vi "utility_panel_single_axis.vi"() -> ()   [LabVIEW 2014]
doc: "This VI is to serve as (1) an example of how one might incorporate the many features of the stepper motor control API into their own application and (2) allows the user to take control of their hardware for demonstration and or troubleshooting purposes. Tips and descriptions have been applied to each control on the interface. Click the HELP button to see more detailed descriptions of each control and their function.\n\nProduced By:\n\nChristopher Lemieux\nKod Integrations, LLC\n4835 Marianne Drive\nMount Airy, MD 21771\nhttp://www.kodintegrations.com\nemail: clemieux@kodintegrations.com\nphone: (240) 687-1288"
uses:
  common/controls/motor_status.ctl
  common/controls/utility_actions.ctl
  classes/Controller/_Controller.lvclass/_Controller.ctl
  common/controls/linear_direction.ctl
  common/controls/movement_item.ctl
  common/controls/axis.ctl
  common/controls/digital_output.ctl
  common/controls/polarity_item.ctl
  common/controls/polarity.ctl
  common/controls/move_mode.ctl
  common/controls/error_actions.ctl
  classes/Controller/_Controller.lvclass
  libraries/common.lvlib
panel:
  in  "help":bool
  out "status (disp)":T1(ring)=enum."CONST"
  out "Current Position (display)":i32=100 min=1 max=5000
  out "date":string
  out "power_led":bool
  in  "on/off":bool
  out "dig_ins":T2
  out "status":T3=enum."CONST"
  in  "jog_to_pos":i32 caption="Jog To Value"
  in  "move_to":bool caption="Jog To..."
  in  "home_neg":bool caption="Home (-)"
  in  "home_pos":bool caption="Home (+)"
  in  "clear":bool caption="Clear Error Codes"
  in  "Tab Control":T4(tab)
  in  "move_mode":enum32{"Abs:", "Inc:"}(radio)
  in  "position_val_set":bool
  out "position_val_actual":i32=100 min=1 max=5000
  in  "position_val_desired":i32
  in  "zero":bool
  in  "demo_start":bool
  in  "pos_3":i32
  in  "pos_2":i32
  in  "pos_1":i32
  in  "accel_set":bool
  out "accel_act":i32=100 min=1 max=5000
  in  "accel":i32=100 min=10 max=1000
  in  "low_speed_set":bool
  in  "high_speed_set":bool
  out "low_speed_act":i32=100 min=100 max=490550
  out "high_speed_act":i32=1 min=1 max=400000
  in  "low_speed":i32=100 min=100 max=490550
  in  "high_speed":i32=50 min=1 max=400000 step=1
  in  "dig_outs":T5
  out "actual_amp":i32
  in  "polarities":T6
  in  "cgh_id":bool
  in  "new_id":string
  in  "run_amp_set":bool
  in  "idle_amp_set":bool
  out "running_amp_act":i32
  out "idle_amp_act":i32
  in  "running_amp":i32=50 min=50 max=2500
  in  "idle_amp":i32=50 min=50 max=2500 step=1
  out "response":string
  out "firmware_ver":string
  out "dev_id":string
  out "prod_id":string
  in  "terminate":bool
  in  "jog_neg":bool caption="Jog (-)"
  in  "jog_pos":bool caption="Jog (+)"
  in  "imm_stop":bool caption="Stop Immediately"
  in  "slow_stop":bool caption="Stop Slowly"
  in  "raw_cmd":string
  in  "write_cmd":bool
  out "error out":errorcluster
  in  "error in (no error)":errorcluster
  # "Firmware:"
  # "Prod ID:"
  # "Dev ID:"
  # "Digital Inputs"
  # "Current Position"
  # "Status:"
  # "Current State"
  # "Mode"
  # "Speed Settings (pps)"
  # "set"
  # "(actual)"
  # "High"
  # "Low"
  # "Acceleration (ms)"
  # "set"
  # "(actual)"
  # "Accel"
  # "Demonstration"
  # "Zero First?"
  # "Position (1)"
  # "Position (2)"
  # "Position (3)"
  # "Position (ticks)"
  # "set"
  # "(actual)"
  # "new"
  # "Current Settings (mA)"
  # "set"
  # "(actual)"
  # "Idle"
  # "Run"
  # "[actual at runtime]"
  # "Polarity Settings:"
  # "Device ID:"
  # "Digital Outputs:"
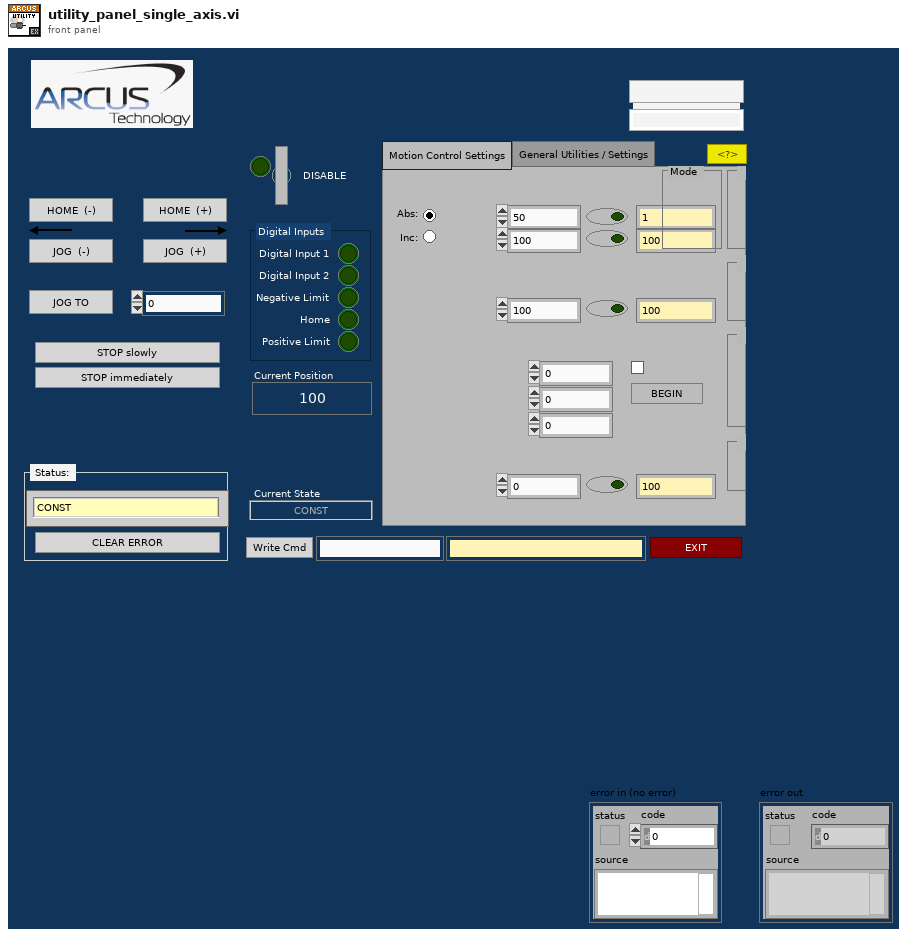
[diagram p1: front panel]
types:
  T1 = enum16{"IDLE", "CONST", "ACCEL", "DECEL", "HOME_SWITCH", "-LIMIT_SWITCH", "+LIMIT_SWITCH", "-LIMIT_ERR", "+LIMIT_ERR", "COMM_TIMEOUT", "ALARM_INPUT", "ALARM_ERROR", "TOC_TIMEOUT_STATUS", "LATCH_INPUT_STATUS", "Z_INDEX_STATUS"}
  T2 = cluster{"Digital Input 1":bool, "Digital Input 2":bool, "Negative Limit":bool, "Home":bool, "Positive Limit":bool}
  T3 = typedef "common.lvlib/motor_status.ctl" = enum16{"IDLE", "CONST", "ACCEL", "DECEL", "HOME_SWITCH", "-LIMIT_SWITCH", "+LIMIT_SWITCH", "-LIMIT_ERR", "+LIMIT_ERR", "COMM_TIMEOUT", "ALARM_INPUT", "ALARM_ERROR", "TOC_TIMEOUT_STATUS", "LATCH_INPUT_STATUS", "Z_INDEX_STATUS"}
  T4 = enum32{"Motion Control Settings", "General Utilities / Settings"}
  T5 = cluster{"Digital Output 1":bool, "Digital Output 2":bool}
  T6 = cluster{"Direction":bool, "Limit":bool, "Home":bool, "Digital Output":bool, "Digital Input":bool, "Enable Output":bool, "Jump On Error":bool}
  T7 = typedef "common.lvlib/utility_actions.ctl" = enum16{"------- unused -------", "about", "checkModel", "clearError", "closeRef", "demo", "getAcceleration", "getActualCurrentVal", "getDeviceId", "getDeviceList", "getDigInputs", "getDigOutputs", "getDriverPowerStatus", "getFirmwareVer", "getHighSpeed", "getIdleCurrent", "getLowSpeed", "getMode", "getPolarity", "getPosition", "getProductId", "getRunCurrent", "getStatus", "homeMotorNeg", "homeMotorPos", "initialize", "jogConstNeg", "jogConstPos", "moveToPos", "openRef", "pause", "powerOFF", "powerON", "processEvents", "rawCmd", "setAcceleration", "setDeviceId", "setDigOutput", "setHighSpeed", "setLowSpeed", "setPolarity", "setPosition", "setRunCurrent", "setIdleCurrent", "setMode", "setTimeOuts", "stopImmediately", "stopSlowly", "storeToFlashMem", "updatePanelItems", "validateDemoPos", "validatePos", "waitUntilDone", "zeroPosition"}
  T8 = typedef "common.lvlib/error_actions.ctl" = enum16{"clearBuff", "closeRef", "nodeErr", "noDeviceInfo", "noDevices", "openRef", "sendReceive", "setTimeouts", "unknown"}
  T9 = typedef "common.lvlib/linear_direction.ctl" = enum16{"POS (+)", "NEG (-)"}
  T10 = typedef "common.lvlib/movement_item.ctl" = cluster{"axis":T11, "target":i32}
  T11 = typedef "common.lvlib/axis.ctl" = enum16{"X", "Y", "Z", "U"}
  T12 = typedef "common.lvlib/digital_output.ctl" = enum16{"DIG_OUT_1", "DIG_OUT_2", "DIG_OUT_3", "DIG_OUT_4", "DIG_OUT_5", "DIG_OUT_6", "DIG_OUT_7", "DIG_OUT_8"}
  T13 = typedef "common.lvlib/polarity_item.ctl" = cluster{"item":T14, "status":bool}
  T14 = typedef "common.lvlib/polarity.ctl" = enum16{"DIRECTION", "LIMIT", "HOME", "DIG_OUT", "DIG_IN", "ENABLE_OUT", "JUMP_ERR", "LATCH", "Z-CHAN_INDEX", "ENCODER_DECODING:1X", "ENCODER_DECODING:2X", "ENCODER_DECODING:4X", "ALARM", "STANDALONE_ERR", "-", "<reserved/nc>"}
  T15 = typedef "common.lvlib/move_mode.ctl" = enum16{"ABSOLUTE", "INCREMENTAL"}
  T16 = typedef "common.lvlib/models.ctl" = enum16{"<unrecognized>", "ACE-SDC", "ACE-SDE", "ACE-SXC", "ACE-SXE", "DMX-CAN", "DMX-J-SA", "DMX-K-SA", "DMX-UMD", "PMX-2ED-SA", "PMX-2EX-SA", "PMX-4CX-SA", "PMX-4EX-SA"}
  T17 = typedef "common.lvlib/digital_input_item.ctl" = cluster{"item":T18, "status":bool}
  T18 = typedef "common.lvlib/digital_input.ctl" = enum16{"DIG_IN_1", "DIG_IN_2", "DIG_IN_3", "DIG_IN_4", "DIG_IN_5", "DIG_IN_6", "DIG_IN_7", "DIG_IN_8", "NEG_LIMIT", "HOME", "POS_LIMIT"}
  T19 = cluster{"[0]":bool, "[1]":bool, "[2]":bool, "[3]":bool, "[4]":bool}
  T20 = typedef "common.lvlib/digital_output_item.ctl" = cluster{"item":T12, "status":bool}
  T21 = cluster{"[0]":bool, "[1]":bool, "[2]":bool, "[3]":bool, "[4]":bool, "[5]":bool, "[6]":bool}
  T22 = typedef "common.lvlib/complete_motor_state.ctl" = cluster{"X":T23, "Y":T23, "Z":T23, "U":T23, "buffer_enabled?":bool, "buffer_start":i32, "buffer_end":i32, "avail_buffer":i32, "move_mode":T15}
  T23 = typedef "common.lvlib/single_axis_state.ctl" = cluster{"motion_state":T3, "other_states":T3[]}
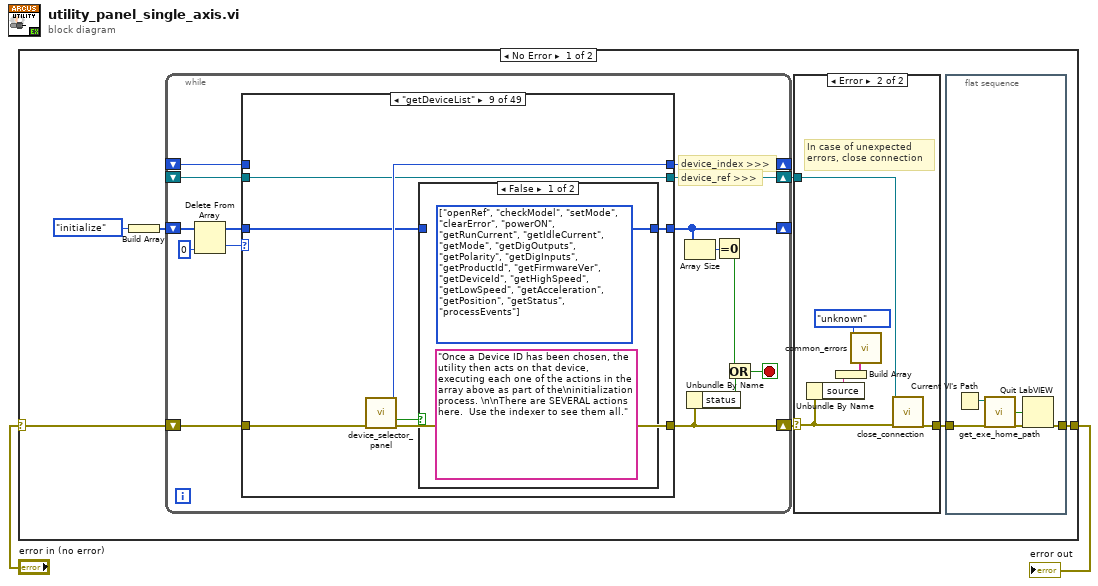
[diagram p0: block diagram]
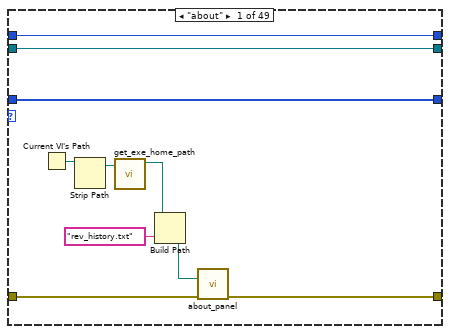
[diagram p3: hidden frame]
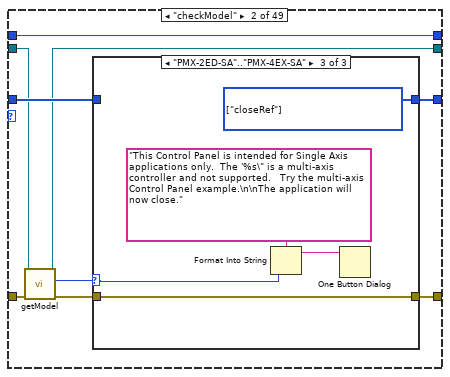
[diagram p4: hidden frame]
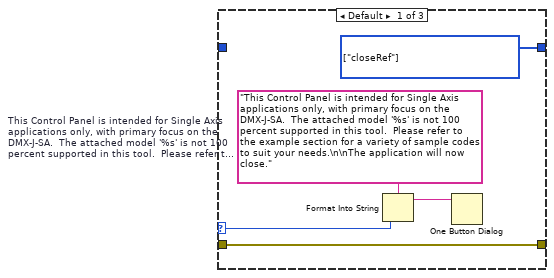
[diagram p5: hidden frame]
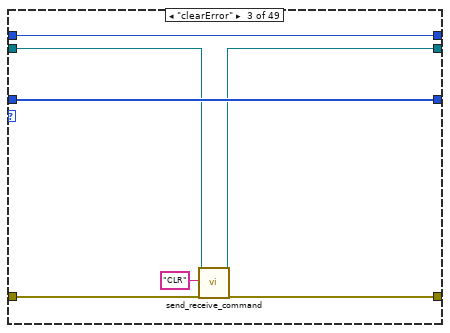
[diagram p7: hidden frame]
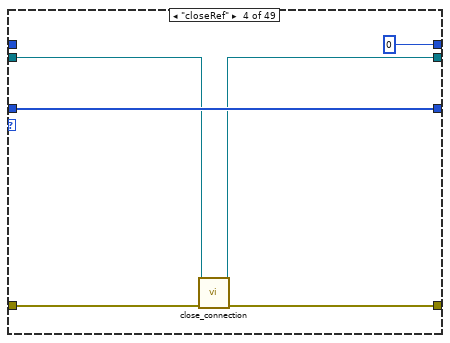
[diagram p8: hidden frame]
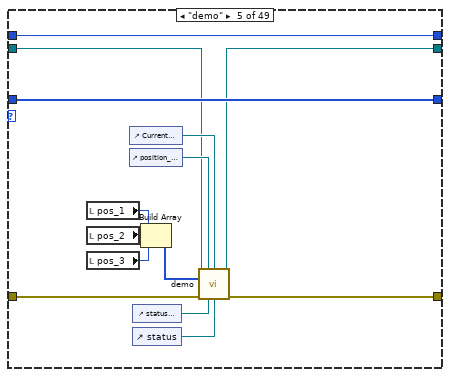
[diagram p9: hidden frame]
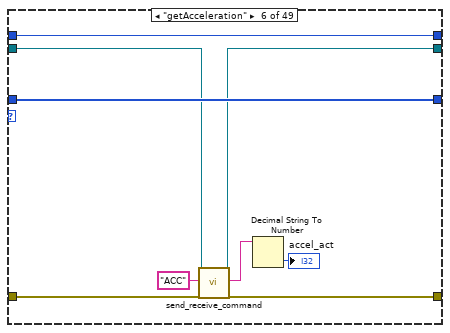
[diagram p10: hidden frame]
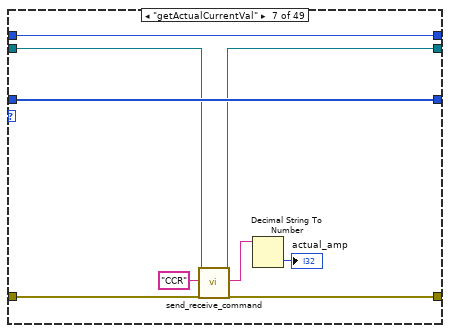
[diagram p11: hidden frame]
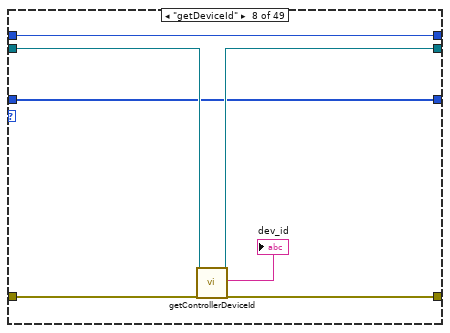
[diagram p12: hidden frame]
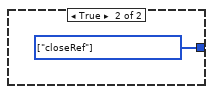
[diagram p13: hidden frame]
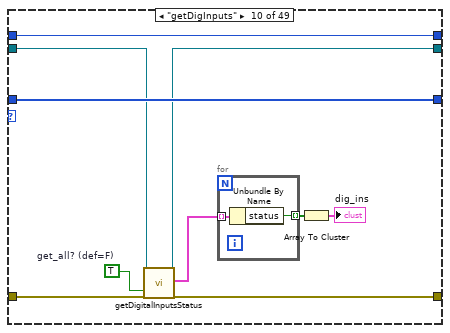
[diagram p14: hidden frame]
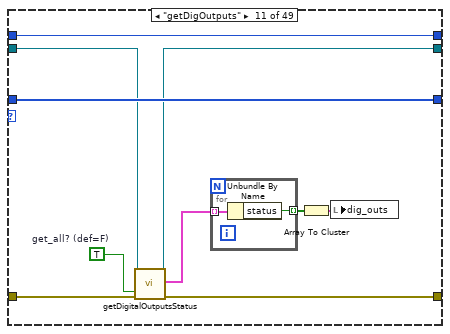
[diagram p15: hidden frame]
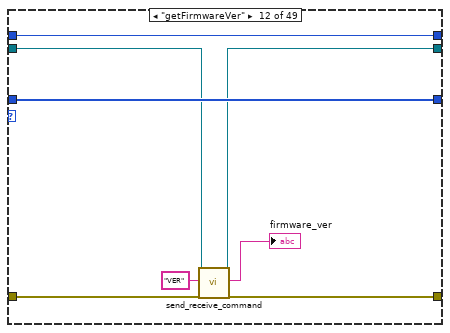
[diagram p16: hidden frame]
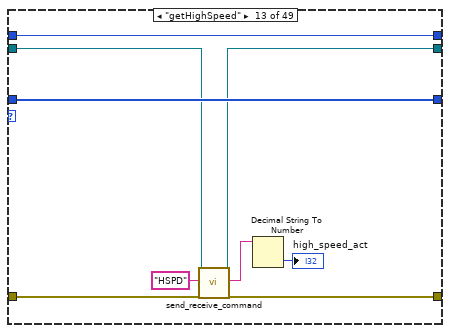
[diagram p17: hidden frame]
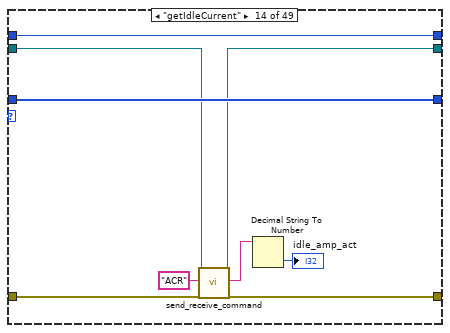
[diagram p18: hidden frame]
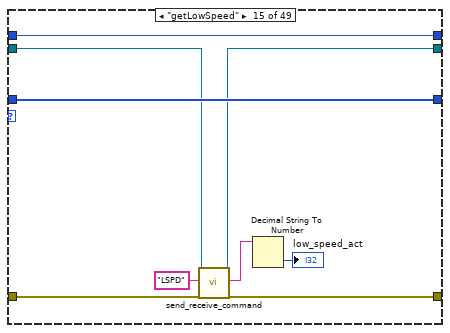
[diagram p19: hidden frame]
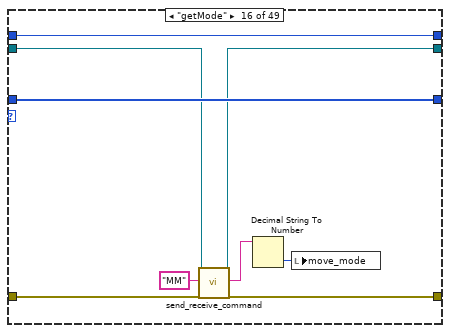
[diagram p20: hidden frame]
diagram:
  n1 = case shown="No Error" "error in (no error)" {
    selector: "error in (no error)" -> [w5 w624]
    tunnel: [w3 w624] -> w1
    frame No Error {
      n2 = Build Array(utility_actions."initialize" ("Enum")) -> (w8:T7[])
      n3 = while {
        shift-right: [w29] -> _
        shift-left: w8 -> [w34]
        shift-right: [w24] -> w7
        shift-left: w5 -> [w30]
        shift-right: [w23] -> w6
        shift-left: _ -> [w22]
        shift-right: [w21] -> _
        shift-left: _ -> [w20]
        stop <- w25 stop-if-true
        # "device_index >>>"
        # "device_ref >>>"
        n4 = Delete From Array(array=w34, index=0) -> (deleted portion=w32:T7, array with subset deleted=w31:T7[])  [unwired: 1 in]
        n5 = case shown="\"getDeviceList\"" w32 {
          tunnel: w31 -> [w44 w51 w72 w78 w88 w101 w110 w111 w119 w136 w148 w158 w167 w176 w185 w194 w203 w212 w220 w229 w237 w245 w253 _ w268 w276 w287 w295 w303 w311 w314 w416 w427 w439 w459 w470 w481 w491 w505 w516 w527 w537 w548 w556 w563 w567 w575 w601 w622]
          tunnel: [w44 w50 w72 w78 w88 w101 w110 w111 w118 w136 w148 w158 w167 w176 w185 w194 w203 w212 w220 w229 w237 w245 w253 w258 w268 w276 w286 w295 w303 w311 w315 w416 w426 w438 w458 w469 w480 w491 w504 w515 w526 w536 w548 w556 w563 w565 w571 w598 w621] -> w29
          tunnel: w30 -> [w41 w52 w70 w77 w87 w99 w108 w117 w124 w131 w146 w156 w165 w174 w183 w192 w201 w210 w218 w227 w235 w242 w250 w260 w265 w273 w284 w294 w300 w308 w318 w417 w425 w437 w455 w468 w479 w487 w503 w514 w525 w532 w546 w554 w561 w564 w572 w599 w620]
          tunnel: [w40 w45 w69 w76 w84 w98 w107 w116 w123 w130 w143 w155 w164 w173 w182 w191 w199 w209 w217 w226 w234 w241 w249 w260 w264 w272 w283 w293 w299 w307 w317 errorcluster {"status"=FALSE, "code"=0, "source"=""} w424 w433 w446 w467 w478 w486 w502 w513 w524 w533 w545 w553 w560 w564 w573 w600 w619] -> w24
          tunnel: [w42 w47 w67 w73 w79 w96 w105 w114 w121 w128 w144 w153 w162 w171 w180 w189 w200 w208 w215 w224 w233 w239 w247 w254 w262 w270 w281 w291 w298 w306 w312 w411 w422 w435 w449 w465 w476 w484 w500 w511 w522 w530 w543 w551 w558 w568 w589 w606 w617] -> w23
          tunnel: w22 -> [w42 w48 w68 w75 w80 w97 w106 w115 w121 w129 w145 w154 w163 w172 w181 w190 w196 w206 w216 w225 w232 w240 w248 w254 w263 w271 w282 _ w296 w304 w312 w412 w423 w436 w454 w466 w477 w485 w501 w512 w523 w531 w544 w552 w559 w568 w589 w606 w618]
          tunnel: [w43 w53 w71 0 ("reference (out)") w89 w100 w109 w113 w122 w135 w147 w157 w166 w175 w184 w193 w202 w211 w219 w228 w236 w244 w252 0 ("index") w267 w275 w288 w292 w302 w310 w313 w413 w428 w440 w460 w471 w482 w492 w506 w517 w528 w538 w547 w555 w562 w569 w590 w607 w623] -> w21
          tunnel: w20 -> [w43 w53 w71 _ w89 w100 w109 w113 _ w135 w147 w157 w166 w175 w184 w193 w202 w211 w219 w228 w236 w244 w252 _ w267 w275 w288 w292 w302 w310 w313 w413 w428 w440 w460 w471 w482 w492 w506 w517 w528 w538 w547 w555 w562 w569 w590 w607 w623]
          frame "about" {
            n6 = Current VI's Path() -> (path=w37:path)
            n7 = Strip Path(path=w37) -> (stripped path=w36:path)  [unwired: 1 out]
            n8 = call "get_exe_home_path.vi"("home_path"=w36) -> ("actual_home_path"=w35:path)  [unwired: 6 in, 1 out]
            n9 = Build Path(base path=w35, name or relative path="rev_history.txt") -> (appended path=w38:path)
            n10 = call "about_panel.vi"("rev_history_filepath"=w38, "error in (no error)"=w41) -> ("error out"=w40:errorcluster)  [unwired: 13 in]
          }
          frame "checkModel" {
            n11 = call "getModel.vi"("error in (no error)"=w52, "reference (in)"=w48) -> ("error out"=w46:errorcluster, "model"=w49:T16, "reference (out)"=w47:refnum<class "_Controller.lvclass">)  [unwired: 7 in]
            n12 = case shown="\"PMX-2ED-SA\"..\"PMX-4EX-SA\"" w49 {
              selector: w49 -> [w55 _ w62]
              tunnel: w51 -> [_ w60 _]
              tunnel: [w54 w60 w64] -> w50
              tunnel: [w58 w59 w65] -> w45
              tunnel: w46 -> [w58 w59 w65]
              frame Default {
                w57 = "This Control Panel is intended for Single Axis applications only, with primary focus on the DMX-J-SA.  The attached model '%s' is not 100 percent supported in this tool.  Please refer to the example section for a variety of sample codes to suit your needs.\n\nThe application will now close."  # This Control Panel is intended for Single Axis applications only, with primary focus on the DMX-J-SA.  The attached model '%s' is not 100 percent supported in this tool.  Please refer to the example section for a variety of sample codes to suit your needs.  The application will now close.
                w54 = T7[] [enum."closeRef"] items=["------- unused -------", "about", "checkModel", "clearError", "closeRef", "demo", "getAcceleration", "getActualCurrentVal", "getDeviceId", "getDeviceList", "getDigInputs", "getDigOutputs", "getDriverPowerStatus", "getFirmwareVer", "getHighSpeed", "getIdleCurrent", "getLowSpeed", "getMode", "getPolarity", "getPosition", "getProductId", "getRunCurrent", "getStatus", "homeMotorNeg", "homeMotorPos", "initialize", "jogConstNeg", "jogConstPos", "moveToPos", "openRef", "pause", "powerOFF", "powerON", "processEvents", "rawCmd", "setAcceleration", "setDeviceId", "setDigOutput", "setHighSpeed", "setLowSpeed", "setPolarity", "setPosition", "setRunCurrent", "setIdleCurrent", "setMode", "setTimeOuts", "stopImmediately", "stopSlowly", "storeToFlashMem", "updatePanelItems", "validateDemoPos", "validatePos", "waitUntilDone", "zeroPosition"] ("actions")
                n13 = Format Into String(format string=w57, w55) -> (resulting string=w56:string)  [unwired: 2 in, 1 out]
                n14 = One Button Dialog(message=w56) -> ()  [unwired: 1 in, 1 out]
              }
              frame "DMX-J-SA" {
                # "fully supported"
              }
              frame "PMX-2ED-SA".."PMX-4EX-SA" {
                w64 = T7[] [enum."closeRef"] items=["------- unused -------", "about", "checkModel", "clearError", "closeRef", "demo", "getAcceleration", "getActualCurrentVal", "getDeviceId", "getDeviceList", "getDigInputs", "getDigOutputs", "getDriverPowerStatus", "getFirmwareVer", "getHighSpeed", "getIdleCurrent", "getLowSpeed", "getMode", "getPolarity", "getPosition", "getProductId", "getRunCurrent", "getStatus", "homeMotorNeg", "homeMotorPos", "initialize", "jogConstNeg", "jogConstPos", "moveToPos", "openRef", "pause", "powerOFF", "powerON", "processEvents", "rawCmd", "setAcceleration", "setDeviceId", "setDigOutput", "setHighSpeed", "setLowSpeed", "setPolarity", "setPosition", "setRunCurrent", "setIdleCurrent", "setMode", "setTimeOuts", "stopImmediately", "stopSlowly", "storeToFlashMem", "updatePanelItems", "validateDemoPos", "validatePos", "waitUntilDone", "zeroPosition"] ("actions")
                n15 = Format Into String(format string="This Control Panel is intended for Single Axis applications only.  The '%s\" is a multi-axis controller and not supported.   Try the multi-axis Control Panel example.\n\nThe application will now close.", w62) -> (resulting string=w61:string)  [unwired: 2 in, 1 out]
                n16 = One Button Dialog(message=w61) -> ()  [unwired: 1 in, 1 out]
              }
            }
          }
          frame "clearError" {
            n17 = call "send_receive_command.vi"("reference (in)"=w68, "ASCII Command (in)"="CLR", "error in (no error)"=w70) -> ("reference (out)"=w67:refnum<class "_Controller.lvclass">, "error out"=w69:errorcluster)  [unwired: 12 in, 3 out]
          }
          frame "closeRef" {
            n18 = call "close_connection.vi"("reference (in)"=w75, "error in (no error)"=w77) -> ("reference (out)"=w73:refnum<class "_Controller.lvclass">, "error out"=w76:errorcluster)  [unwired: 16 in]
          }
          frame "demo" {
            n19 = local read "pos_1"() -> (w91:i32)
            n20 = local read "pos_2"() -> (w90:i32)
            n21 = local read "pos_3"() -> (w92:i32)
            n22 = control-ref of="Current Position (display)"() -> (w83:refnum<vi>)
            n23 = control-ref of="position_val_actual"() -> (w86:refnum<vi>)
            n24 = control-ref of="status (disp)"() -> (w82:refnum<vi>)
            n25 = control-ref of="status"() -> (w81:refnum<vi>)
            n26 = Build Array(w91, w90, w92) -> (w85:i32[])
            n27 = call "demo.vi"("reference (in)"=w80, "position ref"=w86, "position (large) ref"=w83, "positions"=w85, "error in (no error)"=w87, "status (display) ref"=w82, "status ref"=w81) -> ("reference (out)"=w79:refnum<class "_Controller.lvclass">, "error out"=w84:errorcluster)  [unwired: 7 in]
          }
          frame "getAcceleration" {
            n28 = call "send_receive_command.vi"("reference (in)"=w97, "ASCII Command (in)"="ACC", "error in (no error)"=w99) -> ("reference (out)"=w96:refnum<class "_Controller.lvclass">, "response (out)"=w94:string, "error out"=w98:errorcluster)  [unwired: 12 in, 2 out]
            n29 = Decimal String To Number(string=w94) -> (number=→"accel_act":i32)  [unwired: 2 in, 1 out]
          }
          frame "getActualCurrentVal" {
            n30 = call "send_receive_command.vi"("reference (in)"=w106, "ASCII Command (in)"="CCR", "error in (no error)"=w108) -> ("reference (out)"=w105:refnum<class "_Controller.lvclass">, "response (out)"=w104:string, "error out"=w107:errorcluster)  [unwired: 12 in, 2 out]
            n31 = Decimal String To Number(string=w104) -> (number=→"actual_amp":i32)  [unwired: 2 in, 1 out]
          }
          frame "getDeviceId" {
            n32 = call "getControllerDeviceId.vi"("reference (in)"=w115, "error in (no error)"=w117) -> ("reference (out)"=w114:refnum<class "_Controller.lvclass">, "device_id (out)"=→"dev_id":string, "error out"=w116:errorcluster)  [unwired: 15 in]
          }
          frame "getDeviceList" {
            n33 = call "device_selector_panel.vi"("error in (no error)"=w124) -> ("index"=w122:i32, "cancel?"=w120:bool, "error out"=w123:errorcluster)  [unwired: 10 in, 2 out]
            n34 = case shown="False" w120 {
              tunnel: w119 -> [_ _]
              tunnel: [w125 w126] -> w118
              frame False {
                (unwired) "Once a Device ID has been chosen, the utility then acts on that device, executing each one of the actions in the array above as part of the\ninitialization process. \n\nThere are SEVERAL actions here.  Use the indexer to see them all."
                w125 = T7[] [enum."openRef", enum."checkModel", enum."setMode", enum."clearError", enum."powerON", enum."getRunCurrent", enum."getIdleCurrent", enum."getMode", enum."getDigOutputs", enum."getPolarity", enum."getDigInputs", enum."getProductId", enum."getFirmwareVer", enum."getDeviceId", enum."getHighSpeed", enum."getLowSpeed", enum."getAcceleration", enum."getPosition", enum."getStatus", enum."processEvents"] items=["------- unused -------", "about", "checkModel", "clearError", "closeRef", "demo", "getAcceleration", "getActualCurrentVal", "getDeviceId", "getDeviceList", "getDigInputs", "getDigOutputs", "getDriverPowerStatus", "getFirmwareVer", "getHighSpeed", "getIdleCurrent", "getLowSpeed", "getMode", "getPolarity", "getPosition", "getProductId", "getRunCurrent", "getStatus", "homeMotorNeg", "homeMotorPos", "initialize", "jogConstNeg", "jogConstPos", "moveToPos", "openRef", "pause", "powerOFF", "powerON", "processEvents", "rawCmd", "setAcceleration", "setDeviceId", "setDigOutput", "setHighSpeed", "setLowSpeed", "setPolarity", "setPosition", "setRunCurrent", "setIdleCurrent", "setMode", "setTimeOuts", "stopImmediately", "stopSlowly", "storeToFlashMem", "updatePanelItems", "validateDemoPos", "validatePos", "waitUntilDone", "zeroPosition"] ("actions")
              }
              frame True {
                w126 = T7[] [enum."closeRef"] items=["------- unused -------", "about", "checkModel", "clearError", "closeRef", "demo", "getAcceleration", "getActualCurrentVal", "getDeviceId", "getDeviceList", "getDigInputs", "getDigOutputs", "getDriverPowerStatus", "getFirmwareVer", "getHighSpeed", "getIdleCurrent", "getLowSpeed", "getMode", "getPolarity", "getPosition", "getProductId", "getRunCurrent", "getStatus", "homeMotorNeg", "homeMotorPos", "initialize", "jogConstNeg", "jogConstPos", "moveToPos", "openRef", "pause", "powerOFF", "powerON", "processEvents", "rawCmd", "setAcceleration", "setDeviceId", "setDigOutput", "setHighSpeed", "setLowSpeed", "setPolarity", "setPosition", "setRunCurrent", "setIdleCurrent", "setMode", "setTimeOuts", "stopImmediately", "stopSlowly", "storeToFlashMem", "updatePanelItems", "validateDemoPos", "validatePos", "waitUntilDone", "zeroPosition"] ("actions")
              }
            }
          }
          frame "getDigInputs" {
            w132 = TRUE  # get_all? (def=F)
            n35 = call "getDigitalInputsStatus.vi"("Controller in"=w129, "get_all? (def=F)"=w132, "error in (no error)"=w131) -> ("Controller out"=w128:refnum<class "_Controller.lvclass">, "di_items"=w127:T17[], "error out"=w130:errorcluster)  [unwired: 12 in, 2 out]
            n36 = for {
              tunnel: w127 -> [w138] mode=indexing
              tunnel: [w137] -> w134 mode=indexing
              n37 = Unbundle By Name(w138) -> ("status"=w137:bool)
            }
            n38 = Array To Cluster(array=w134) -> (cluster=→"dig_ins":T19)
          }
          frame "getDigOutputs" {
            w139 = TRUE  # get_all? (def=F)
            n39 = call "getDigitalOutputsStatus.vi"("Controller in"=w145, "get_all? (def=F)"=w139, "error in (no error)"=w146) -> ("Controller out"=w144:refnum<class "_Controller.lvclass">, "do_items"=w142:T20[], "error out"=w143:errorcluster)  [unwired: 12 in, 2 out]
            n40 = for {
              tunnel: w142 -> [w150] mode=indexing
              tunnel: [w149] -> w141 mode=indexing
              n41 = Unbundle By Name(w150) -> ("status"=w149:bool)
            }
            n42 = Array To Cluster(array=w141) -> (cluster=w140:cluster{"[0]":bool, "[1]":bool})
            n43 = local write "dig_outs"(w140) -> ()
          }
          frame "getFirmwareVer" {
            n44 = call "send_receive_command.vi"("reference (in)"=w154, "ASCII Command (in)"="VER", "error in (no error)"=w156) -> ("reference (out)"=w153:refnum<class "_Controller.lvclass">, "response (out)"=→"firmware_ver":string, "error out"=w155:errorcluster)  [unwired: 12 in, 2 out]
          }
          frame "getHighSpeed" {
            n45 = call "send_receive_command.vi"("reference (in)"=w163, "ASCII Command (in)"="HSPD", "error in (no error)"=w165) -> ("reference (out)"=w162:refnum<class "_Controller.lvclass">, "response (out)"=w161:string, "error out"=w164:errorcluster)  [unwired: 12 in, 2 out]
            n46 = Decimal String To Number(string=w161) -> (number=→"high_speed_act":i32)  [unwired: 2 in, 1 out]
          }
          frame "getIdleCurrent" {
            n47 = call "send_receive_command.vi"("reference (in)"=w172, "ASCII Command (in)"="ACR", "error in (no error)"=w174) -> ("reference (out)"=w171:refnum<class "_Controller.lvclass">, "response (out)"=w170:string, "error out"=w173:errorcluster)  [unwired: 12 in, 2 out]
            n48 = Decimal String To Number(string=w170) -> (number=→"idle_amp_act":i32)  [unwired: 2 in, 1 out]
          }
          frame "getLowSpeed" {
            n49 = call "send_receive_command.vi"("reference (in)"=w181, "ASCII Command (in)"="LSPD", "error in (no error)"=w183) -> ("reference (out)"=w180:refnum<class "_Controller.lvclass">, "response (out)"=w179:string, "error out"=w182:errorcluster)  [unwired: 12 in, 2 out]
            n50 = Decimal String To Number(string=w179) -> (number=→"low_speed_act":i32)  [unwired: 2 in, 1 out]
          }
          frame "getMode" {
            n51 = call "send_receive_command.vi"("reference (in)"=w190, "ASCII Command (in)"="MM", "error in (no error)"=w192) -> ("reference (out)"=w189:refnum<class "_Controller.lvclass">, "response (out)"=w188:string, "error out"=w191:errorcluster)  [unwired: 12 in, 2 out]
            n52 = Decimal String To Number(string=w188) -> (number=w187:i32)  [unwired: 2 in, 1 out]
            n53 = local write "move_mode"(w187) -> ()
          }
          frame "getPolarity" {
            n54 = call-dynamic "getPolarity.vi"("Controller in"=w196, "error in (no error)"=w201) -> ("Controller out"=w200:refnum<class "_Controller.lvclass">, "polarity_items (out)"=w195:T13[], "error out"=w199:errorcluster)  [unwired: 15 in]
            n55 = for {
              tunnel: w195 -> [w205] mode=indexing
              tunnel: [w204] -> w198 mode=indexing
              n56 = Unbundle By Name(w205) -> ("status"=w204:bool)
            }
            n57 = Array To Cluster(array=w198) -> (cluster=w197:T21)
            n58 = local write "polarities"(w197) -> ()
          }
          frame "getPosition" {
            n59 = call-dynamic "getCurrentPosition.vi"("reference (in)"=w206, "error in (no error)"=w210) -> ("reference (out)"=w208:refnum<class "_Controller.lvclass">, "current_position (units)"=→"position_val_actual" →"Current Position (display)":i32, "error out"=w209:errorcluster)  [unwired: 15 in]
          }
          frame "getProductId" {
            n60 = call "send_receive_command.vi"("reference (in)"=w216, "ASCII Command (in)"="ID", "error in (no error)"=w218) -> ("reference (out)"=w215:refnum<class "_Controller.lvclass">, "response (out)"=→"prod_id":string, "error out"=w217:errorcluster)  [unwired: 12 in, 2 out]
          }
          frame "getRunCurrent" {
            n61 = call "send_receive_command.vi"("reference (in)"=w225, "ASCII Command (in)"="CUR", "error in (no error)"=w227) -> ("reference (out)"=w224:refnum<class "_Controller.lvclass">, "response (out)"=w223:string, "error out"=w226:errorcluster)  [unwired: 12 in, 2 out]
            n62 = Decimal String To Number(string=w223) -> (number=→"running_amp_act":i32)  [unwired: 2 in, 1 out]
          }
          frame "getStatus" {
            n63 = call-dynamic "getStatus.vi"("reference (in)"=w232, "error in (no error)"=w235) -> ("reference (out)"=w233:refnum<class "_Controller.lvclass">, "full_state"=w231:T22, "error out"=w234:errorcluster)  [unwired: 14 in, 1 out]
            n64 = Unbundle By Name(w231) -> ("X.motion_state"=→"status" →"status (disp)":T3)
          }
          frame "homeMotorNeg" {
            w243 = u8 2 ("Disabled")
            n65 = call-dynamic "goToHome.vi"("Controller in"=w240, "dir"=linear_direction."NEG (-)", "error in (no error)"=w242) -> ("Controller out"=w239:refnum<class "_Controller.lvclass">, "error out"=w241:errorcluster)  [unwired: 13 in, 2 out]
            n66 = property on="home_neg" class="Bool"("Disabled"=w243) -> ()  [unwired: 2 in, 2 out]
            n67 = property on="home_pos" class="Bool"("Disabled"=w243) -> ()  [unwired: 2 in, 2 out]
            n68 = property on="move_to" class="Bool"("Disabled"=w243) -> ()  [unwired: 2 in, 2 out]
            n69 = property on="jog_pos" class="Bool"("Disabled"=w243) -> ()  [unwired: 2 in, 2 out]
            n70 = property on="jog_neg" class="Bool"("Disabled"=w243) -> ()  [unwired: 2 in, 2 out]
          }
          frame "homeMotorPos" {
            w251 = u8 2 ("Disabled")
            n71 = call-dynamic "goToHome.vi"("Controller in"=w248, "dir"=linear_direction."POS (+)", "error in (no error)"=w250) -> ("Controller out"=w247:refnum<class "_Controller.lvclass">, "error out"=w249:errorcluster)  [unwired: 13 in, 2 out]
            n72 = property on="home_neg" class="Bool"("Disabled"=w251) -> ()  [unwired: 2 in, 2 out]
            n73 = property on="home_pos" class="Bool"("Disabled"=w251) -> ()  [unwired: 2 in, 2 out]
            n74 = property on="move_to" class="Bool"("Disabled"=w251) -> ()  [unwired: 2 in, 2 out]
            n75 = property on="jog_pos" class="Bool"("Disabled"=w251) -> ()  [unwired: 2 in, 2 out]
            n76 = property on="jog_neg" class="Bool"("Disabled"=w251) -> ()  [unwired: 2 in, 2 out]
          }
          frame "initialize", Default {
            w255 = u8 0 ("Disabled")
            w258 = T7[] [enum."getDeviceList"] items=["------- unused -------", "about", "checkModel", "clearError", "closeRef", "demo", "getAcceleration", "getActualCurrentVal", "getDeviceId", "getDeviceList", "getDigInputs", "getDigOutputs", "getDriverPowerStatus", "getFirmwareVer", "getHighSpeed", "getIdleCurrent", "getLowSpeed", "getMode", "getPolarity", "getPosition", "getProductId", "getRunCurrent", "getStatus", "homeMotorNeg", "homeMotorPos", "initialize", "jogConstNeg", "jogConstPos", "moveToPos", "openRef", "pause", "powerOFF", "powerON", "processEvents", "rawCmd", "setAcceleration", "setDeviceId", "setDigOutput", "setHighSpeed", "setLowSpeed", "setPolarity", "setPosition", "setRunCurrent", "setIdleCurrent", "setMode", "setTimeOuts", "stopImmediately", "stopSlowly", "storeToFlashMem", "updatePanelItems", "validateDemoPos", "validatePos", "waitUntilDone", "zeroPosition"] ("actions")
            w256 = ""
            w259 = FALSE
            n77 = property on="home_neg" class="Bool"("Disabled"=w255) -> ()  [unwired: 2 in, 2 out]
            n78 = property on="home_pos" class="Bool"("Disabled"=w255) -> ()  [unwired: 2 in, 2 out]
            n79 = property on="move_to" class="Bool"("Disabled"=w255) -> ()  [unwired: 2 in, 2 out]
            n80 = property on="jog_pos" class="Bool"("Disabled"=w255) -> ()  [unwired: 2 in, 2 out]
            n81 = property on="jog_neg" class="Bool"("Disabled"=w255) -> ()  [unwired: 2 in, 2 out]
            n82 = local write "on/off"(w259) -> ()
            n83 = local write "power_led"(w259) -> ()
            n84 = local write "new_id"(w256) -> ()
            n85 = local write "raw_cmd"(w256) -> ()
            n86 = local write "response"(w256) -> ()
          }
          frame "jogConstNeg" {
            w266 = u8 2 ("Disabled")
            n87 = call-dynamic "jogMotor.vi"("Controller in"=w263, "dir"=linear_direction."NEG (-)", "error in (no error)"=w265) -> ("Controller out"=w262:refnum<class "_Controller.lvclass">, "error out"=w264:errorcluster)  [unwired: 13 in, 2 out]
            n88 = property on="home_neg" class="Bool"("Disabled"=w266) -> ()  [unwired: 2 in, 2 out]
            n89 = property on="home_pos" class="Bool"("Disabled"=w266) -> ()  [unwired: 2 in, 2 out]
            n90 = property on="move_to" class="Bool"("Disabled"=w266) -> ()  [unwired: 2 in, 2 out]
            n91 = property on="jog_pos" class="Bool"("Disabled"=w266) -> ()  [unwired: 2 in, 2 out]
            n92 = property on="jog_neg" class="Bool"("Disabled"=w266) -> ()  [unwired: 2 in, 2 out]
          }
          frame "jogConstPos" {
            w274 = u8 2 ("Disabled")
            n93 = call-dynamic "jogMotor.vi"("Controller in"=w271, "dir"=linear_direction."POS (+)", "error in (no error)"=w273) -> ("Controller out"=w270:refnum<class "_Controller.lvclass">, "error out"=w272:errorcluster)  [unwired: 13 in, 2 out]
            n94 = property on="home_neg" class="Bool"("Disabled"=w274) -> ()  [unwired: 2 in, 2 out]
            n95 = property on="home_pos" class="Bool"("Disabled"=w274) -> ()  [unwired: 2 in, 2 out]
            n96 = property on="move_to" class="Bool"("Disabled"=w274) -> ()  [unwired: 2 in, 2 out]
            n97 = property on="jog_pos" class="Bool"("Disabled"=w274) -> ()  [unwired: 2 in, 2 out]
            n98 = property on="jog_neg" class="Bool"("Disabled"=w274) -> ()  [unwired: 2 in, 2 out]
          }
          frame "moveToPos" {
            n99 = local read "jog_to_pos"() -> (w279:i32)
            n100 = Bundle By Name(cluster=T10 {"axis"=enum."X", "target"=0} ("item"), "target"=w279) -> (w278:T10)
            n101 = Build Array(w278) -> (w277:T10[])
            n102 = call-dynamic "moveToPosition.vi"("Controller in"=w282, "target(s) (in)"=w277, "error in (no error)"=w284) -> ("Controller out"=w281:refnum<class "_Controller.lvclass">, "error out"=w283:errorcluster)  [unwired: 13 in, 2 out]
            n103 = Build Array (concatenate)(utility_actions."getPosition" ("Enum"), w287) -> (w286:T7[])
          }
          frame "openRef" {
            w289 = 1000  # write_timeout (ms); def=1000
            w290 = 1000  # read_timeout (ms); def=1000
            n104 = call "initialize.vi"("device_index (in) [0=def]"=w292, "read_timeout (ms); def=1000"=w290, "write_timeout (ms); def=1000"=w289, "error in (no error)"=w294) -> ("reference (out)"=w291:refnum<class "_Controller.lvclass">, "error out"=w293:errorcluster)  [unwired: 14 in]
          }
          frame "powerOFF" {
            w297 = FALSE
            w301 = FALSE  # state (def=OFF)
            # "in the event this \ncase is triggered by\nsomething other \nthan the toggle"
            n105 = call-dynamic "setEnabledState.vi"("Controller in"=w296, "state (for single-axis applications only) - (def = DISABLED)"=w301, "error in (no error)"=w300) -> ("Controller out"=w298:refnum<class "_Controller.lvclass">, "error out"=w299:errorcluster)  [unwired: 13 in, 2 out]
            n106 = local write "power_led"(w297) -> ()
            n107 = local write "on/off"(w297) -> ()
          }
          frame "powerON" {
            w305 = TRUE
            w309 = TRUE  # state (def=OFF)
            # "in the event this \ncase is triggered by\nsomething other \nthan the toggle"
            n108 = call-dynamic "setEnabledState.vi"("Controller in"=w304, "state (for single-axis applications only) - (def = DISABLED)"=w309, "error in (no error)"=w308) -> ("Controller out"=w306:refnum<class "_Controller.lvclass">, "error out"=w307:errorcluster)  [unwired: 13 in, 2 out]
            n109 = local write "power_led"(w305) -> ()
            n110 = local write "on/off"(w305) -> ()
          }
          frame "processEvents" {
            n111 = event shown="[20] Menu Selection (User)" {
              selector: _ -> [_ _ _ _ _ _ _ _ _ _ _ _ _ _ _ _ _ _ _ _ _ _ _ _ _]
              dyn-events: _ -> [_ _ _ _ _ _ _ _ _ _ _ _ _ _ _ _ _ _ _ _ _ _ _ _ _]
              timeout: 20 -> [_ _ _ _ _ _ _ _ _ _ _ _ _ _ _ _ _ _ _ _ _ _ _ _ _]
              tunnel: [w322 w324 w326 w328 w330 w332 w334 w337 w341 w343 w352 w356 w358 w360 w362 w364 w366 w368 w371 w375 w376 w401 w405 w407 w409] -> w317
              tunnel: w318 -> [w322 w324 w326 w328 w330 w332 w334 w337 w341 w343 w352 w356 w358 w360 w362 w364 w366 w368 w371 w375 w376 w401 w405 w407 w409]
              tunnel: [w321 w323 w325 w327 w329 w331 w333 w336 w340 w342 w351 w355 w357 w359 w361 w363 w365 w367 w370 w374 w377 w400 w404 w406 w408] -> w315
              tunnel: w314 -> [_ _ _ _ _ _ _ _ _ _ _ _ _ _ _ _ _ _ _ _ _ _ _ _ _]
              event Timeout {
                w321 = T7[] [enum."updatePanelItems", enum."getDigInputs", enum."getPosition", enum."getStatus", enum."getActualCurrentVal", enum."processEvents"] items=["------- unused -------", "about", "checkModel", "clearError", "closeRef", "demo", "getAcceleration", "getActualCurrentVal", "getDeviceId", "getDeviceList", "getDigInputs", "getDigOutputs", "getDriverPowerStatus", "getFirmwareVer", "getHighSpeed", "getIdleCurrent", "getLowSpeed", "getMode", "getPolarity", "getPosition", "getProductId", "getRunCurrent", "getStatus", "homeMotorNeg", "homeMotorPos", "initialize", "jogConstNeg", "jogConstPos", "moveToPos", "openRef", "pause", "powerOFF", "powerON", "processEvents", "rawCmd", "setAcceleration", "setDeviceId", "setDigOutput", "setHighSpeed", "setLowSpeed", "setPolarity", "setPosition", "setRunCurrent", "setIdleCurrent", "setMode", "setTimeOuts", "stopImmediately", "stopSlowly", "storeToFlashMem", "updatePanelItems", "validateDemoPos", "validatePos", "waitUntilDone", "zeroPosition"] ("actions")
                n112 = event-data() -> ()  [unwired: 1 in, 2 out]
                n113 = Format Date/Time String(time format string (%c)="%B %d, %Y - %H:%M:%S") -> (date/time string=→"date":string)  [unwired: 2 in]
              }
              event "write_cmd": Value Change {
                w323 = T7[] [enum."rawCmd", enum."processEvents"] items=["------- unused -------", "about", "checkModel", "clearError", "closeRef", "demo", "getAcceleration", "getActualCurrentVal", "getDeviceId", "getDeviceList", "getDigInputs", "getDigOutputs", "getDriverPowerStatus", "getFirmwareVer", "getHighSpeed", "getIdleCurrent", "getLowSpeed", "getMode", "getPolarity", "getPosition", "getProductId", "getRunCurrent", "getStatus", "homeMotorNeg", "homeMotorPos", "initialize", "jogConstNeg", "jogConstPos", "moveToPos", "openRef", "pause", "powerOFF", "powerON", "processEvents", "rawCmd", "setAcceleration", "setDeviceId", "setDigOutput", "setHighSpeed", "setLowSpeed", "setPolarity", "setPosition", "setRunCurrent", "setIdleCurrent", "setMode", "setTimeOuts", "stopImmediately", "stopSlowly", "storeToFlashMem", "updatePanelItems", "validateDemoPos", "validatePos", "waitUntilDone", "zeroPosition"] ("actions")
                n114 = event-data() -> ()  [unwired: 1 in, 6 out]
              }
              event "slow_stop": Value Change {
                w325 = T7[] [enum."stopSlowly", enum."processEvents"] items=["------- unused -------", "about", "checkModel", "clearError", "closeRef", "demo", "getAcceleration", "getActualCurrentVal", "getDeviceId", "getDeviceList", "getDigInputs", "getDigOutputs", "getDriverPowerStatus", "getFirmwareVer", "getHighSpeed", "getIdleCurrent", "getLowSpeed", "getMode", "getPolarity", "getPosition", "getProductId", "getRunCurrent", "getStatus", "homeMotorNeg", "homeMotorPos", "initialize", "jogConstNeg", "jogConstPos", "moveToPos", "openRef", "pause", "powerOFF", "powerON", "processEvents", "rawCmd", "setAcceleration", "setDeviceId", "setDigOutput", "setHighSpeed", "setLowSpeed", "setPolarity", "setPosition", "setRunCurrent", "setIdleCurrent", "setMode", "setTimeOuts", "stopImmediately", "stopSlowly", "storeToFlashMem", "updatePanelItems", "validateDemoPos", "validatePos", "waitUntilDone", "zeroPosition"] ("actions")
                n115 = event-data() -> ()  [unwired: 1 in, 6 out]
              }
              event "imm_stop": Value Change {
                w327 = T7[] [enum."stopImmediately", enum."processEvents"] items=["------- unused -------", "about", "checkModel", "clearError", "closeRef", "demo", "getAcceleration", "getActualCurrentVal", "getDeviceId", "getDeviceList", "getDigInputs", "getDigOutputs", "getDriverPowerStatus", "getFirmwareVer", "getHighSpeed", "getIdleCurrent", "getLowSpeed", "getMode", "getPolarity", "getPosition", "getProductId", "getRunCurrent", "getStatus", "homeMotorNeg", "homeMotorPos", "initialize", "jogConstNeg", "jogConstPos", "moveToPos", "openRef", "pause", "powerOFF", "powerON", "processEvents", "rawCmd", "setAcceleration", "setDeviceId", "setDigOutput", "setHighSpeed", "setLowSpeed", "setPolarity", "setPosition", "setRunCurrent", "setIdleCurrent", "setMode", "setTimeOuts", "stopImmediately", "stopSlowly", "storeToFlashMem", "updatePanelItems", "validateDemoPos", "validatePos", "waitUntilDone", "zeroPosition"] ("actions")
                n116 = event-data() -> ()  [unwired: 1 in, 6 out]
              }
              event "jog_pos": Value Change {
                w329 = T7[] [enum."jogConstPos", enum."processEvents"] items=["------- unused -------", "about", "checkModel", "clearError", "closeRef", "demo", "getAcceleration", "getActualCurrentVal", "getDeviceId", "getDeviceList", "getDigInputs", "getDigOutputs", "getDriverPowerStatus", "getFirmwareVer", "getHighSpeed", "getIdleCurrent", "getLowSpeed", "getMode", "getPolarity", "getPosition", "getProductId", "getRunCurrent", "getStatus", "homeMotorNeg", "homeMotorPos", "initialize", "jogConstNeg", "jogConstPos", "moveToPos", "openRef", "pause", "powerOFF", "powerON", "processEvents", "rawCmd", "setAcceleration", "setDeviceId", "setDigOutput", "setHighSpeed", "setLowSpeed", "setPolarity", "setPosition", "setRunCurrent", "setIdleCurrent", "setMode", "setTimeOuts", "stopImmediately", "stopSlowly", "storeToFlashMem", "updatePanelItems", "validateDemoPos", "validatePos", "waitUntilDone", "zeroPosition"] ("actions")
                n117 = event-data() -> ()  [unwired: 1 in, 6 out]
              }
              event "jog_neg": Value Change {
                w331 = T7[] [enum."jogConstNeg", enum."processEvents"] items=["------- unused -------", "about", "checkModel", "clearError", "closeRef", "demo", "getAcceleration", "getActualCurrentVal", "getDeviceId", "getDeviceList", "getDigInputs", "getDigOutputs", "getDriverPowerStatus", "getFirmwareVer", "getHighSpeed", "getIdleCurrent", "getLowSpeed", "getMode", "getPolarity", "getPosition", "getProductId", "getRunCurrent", "getStatus", "homeMotorNeg", "homeMotorPos", "initialize", "jogConstNeg", "jogConstPos", "moveToPos", "openRef", "pause", "powerOFF", "powerON", "processEvents", "rawCmd", "setAcceleration", "setDeviceId", "setDigOutput", "setHighSpeed", "setLowSpeed", "setPolarity", "setPosition", "setRunCurrent", "setIdleCurrent", "setMode", "setTimeOuts", "stopImmediately", "stopSlowly", "storeToFlashMem", "updatePanelItems", "validateDemoPos", "validatePos", "waitUntilDone", "zeroPosition"] ("actions")
                n118 = event-data() -> ()  [unwired: 1 in, 6 out]
              }
              event "terminate": Value Change {
                w333 = T7[] [enum."powerOFF", enum."closeRef"] items=["------- unused -------", "about", "checkModel", "clearError", "closeRef", "demo", "getAcceleration", "getActualCurrentVal", "getDeviceId", "getDeviceList", "getDigInputs", "getDigOutputs", "getDriverPowerStatus", "getFirmwareVer", "getHighSpeed", "getIdleCurrent", "getLowSpeed", "getMode", "getPolarity", "getPosition", "getProductId", "getRunCurrent", "getStatus", "homeMotorNeg", "homeMotorPos", "initialize", "jogConstNeg", "jogConstPos", "moveToPos", "openRef", "pause", "powerOFF", "powerON", "processEvents", "rawCmd", "setAcceleration", "setDeviceId", "setDigOutput", "setHighSpeed", "setLowSpeed", "setPolarity", "setPosition", "setRunCurrent", "setIdleCurrent", "setMode", "setTimeOuts", "stopImmediately", "stopSlowly", "storeToFlashMem", "updatePanelItems", "validateDemoPos", "validatePos", "waitUntilDone", "zeroPosition"] ("actions")
                n119 = event-data() -> ()  [unwired: 1 in, 6 out]
              }
              event "on/off": Value Change {
                n120 = event-data() -> ("NewVal"=w335:bool)  [unwired: 1 in, 5 out]
                "power_led" <- w335
                n121 = case shown="False" w335 {
                  tunnel: [w338 w339] -> w336
                  frame True {
                    w338 = T7[] [enum."powerON", enum."processEvents"] items=["------- unused -------", "about", "checkModel", "clearError", "closeRef", "demo", "getAcceleration", "getActualCurrentVal", "getDeviceId", "getDeviceList", "getDigInputs", "getDigOutputs", "getDriverPowerStatus", "getFirmwareVer", "getHighSpeed", "getIdleCurrent", "getLowSpeed", "getMode", "getPolarity", "getPosition", "getProductId", "getRunCurrent", "getStatus", "homeMotorNeg", "homeMotorPos", "initialize", "jogConstNeg", "jogConstPos", "moveToPos", "openRef", "pause", "powerOFF", "powerON", "processEvents", "rawCmd", "setAcceleration", "setDeviceId", "setDigOutput", "setHighSpeed", "setLowSpeed", "setPolarity", "setPosition", "setRunCurrent", "setIdleCurrent", "setMode", "setTimeOuts", "stopImmediately", "stopSlowly", "storeToFlashMem", "updatePanelItems", "validateDemoPos", "validatePos", "waitUntilDone", "zeroPosition"] ("actions")
                  }
                  frame False {
                    w339 = T7[] [enum."powerOFF", enum."processEvents"] items=["------- unused -------", "about", "checkModel", "clearError", "closeRef", "demo", "getAcceleration", "getActualCurrentVal", "getDeviceId", "getDeviceList", "getDigInputs", "getDigOutputs", "getDriverPowerStatus", "getFirmwareVer", "getHighSpeed", "getIdleCurrent", "getLowSpeed", "getMode", "getPolarity", "getPosition", "getProductId", "getRunCurrent", "getStatus", "homeMotorNeg", "homeMotorPos", "initialize", "jogConstNeg", "jogConstPos", "moveToPos", "openRef", "pause", "powerOFF", "powerON", "processEvents", "rawCmd", "setAcceleration", "setDeviceId", "setDigOutput", "setHighSpeed", "setLowSpeed", "setPolarity", "setPosition", "setRunCurrent", "setIdleCurrent", "setMode", "setTimeOuts", "stopImmediately", "stopSlowly", "storeToFlashMem", "updatePanelItems", "validateDemoPos", "validatePos", "waitUntilDone", "zeroPosition"] ("actions")
                  }
                }
              }
              event "idle_amp_set": Value Change {
                w340 = T7[] [enum."setIdleCurrent", enum."processEvents"] items=["------- unused -------", "about", "checkModel", "clearError", "closeRef", "demo", "getAcceleration", "getActualCurrentVal", "getDeviceId", "getDeviceList", "getDigInputs", "getDigOutputs", "getDriverPowerStatus", "getFirmwareVer", "getHighSpeed", "getIdleCurrent", "getLowSpeed", "getMode", "getPolarity", "getPosition", "getProductId", "getRunCurrent", "getStatus", "homeMotorNeg", "homeMotorPos", "initialize", "jogConstNeg", "jogConstPos", "moveToPos", "openRef", "pause", "powerOFF", "powerON", "processEvents", "rawCmd", "setAcceleration", "setDeviceId", "setDigOutput", "setHighSpeed", "setLowSpeed", "setPolarity", "setPosition", "setRunCurrent", "setIdleCurrent", "setMode", "setTimeOuts", "stopImmediately", "stopSlowly", "storeToFlashMem", "updatePanelItems", "validateDemoPos", "validatePos", "waitUntilDone", "zeroPosition"] ("actions")
                n122 = event-data() -> ()  [unwired: 1 in, 6 out]
              }
              event "run_amp_set": Value Change {
                w342 = T7[] [enum."setRunCurrent", enum."processEvents"] items=["------- unused -------", "about", "checkModel", "clearError", "closeRef", "demo", "getAcceleration", "getActualCurrentVal", "getDeviceId", "getDeviceList", "getDigInputs", "getDigOutputs", "getDriverPowerStatus", "getFirmwareVer", "getHighSpeed", "getIdleCurrent", "getLowSpeed", "getMode", "getPolarity", "getPosition", "getProductId", "getRunCurrent", "getStatus", "homeMotorNeg", "homeMotorPos", "initialize", "jogConstNeg", "jogConstPos", "moveToPos", "openRef", "pause", "powerOFF", "powerON", "processEvents", "rawCmd", "setAcceleration", "setDeviceId", "setDigOutput", "setHighSpeed", "setLowSpeed", "setPolarity", "setPosition", "setRunCurrent", "setIdleCurrent", "setMode", "setTimeOuts", "stopImmediately", "stopSlowly", "storeToFlashMem", "updatePanelItems", "validateDemoPos", "validatePos", "waitUntilDone", "zeroPosition"] ("actions")
                n123 = event-data() -> ()  [unwired: 1 in, 6 out]
              }
              event "cgh_id": Value Change {
                n124 = event-data() -> ()  [unwired: 1 in, 6 out]
                n125 = local read "new_id"() -> (w348:string)
                n126 = local read "dev_id"() -> (w349:string)
                n127 = Format Into String(format string="Are you sure you want to change the\nDevice ID from '%s' to '%s'?", w349, w348) -> (resulting string=w347:string)  [unwired: 2 in, 1 out]
                n128 = Two Button Dialog(message=w347, 1:"Cancel" ("T button name (\"OK\")"), 2:"Yes" ("T button name (\"OK\")")) -> (T button?=w344:bool)
                n129 = case shown="False" w344 {
                  tunnel: [w353 w354] -> w351
                  frame True {
                    w353 = T7[] [enum."setDeviceId", enum."processEvents"] items=["------- unused -------", "about", "checkModel", "clearError", "closeRef", "demo", "getAcceleration", "getActualCurrentVal", "getDeviceId", "getDeviceList", "getDigInputs", "getDigOutputs", "getDriverPowerStatus", "getFirmwareVer", "getHighSpeed", "getIdleCurrent", "getLowSpeed", "getMode", "getPolarity", "getPosition", "getProductId", "getRunCurrent", "getStatus", "homeMotorNeg", "homeMotorPos", "initialize", "jogConstNeg", "jogConstPos", "moveToPos", "openRef", "pause", "powerOFF", "powerON", "processEvents", "rawCmd", "setAcceleration", "setDeviceId", "setDigOutput", "setHighSpeed", "setLowSpeed", "setPolarity", "setPosition", "setRunCurrent", "setIdleCurrent", "setMode", "setTimeOuts", "stopImmediately", "stopSlowly", "storeToFlashMem", "updatePanelItems", "validateDemoPos", "validatePos", "waitUntilDone", "zeroPosition"] ("actions")
                  }
                  frame False {
                    w354 = T7[] [enum."processEvents"] items=["------- unused -------", "about", "checkModel", "clearError", "closeRef", "demo", "getAcceleration", "getActualCurrentVal", "getDeviceId", "getDeviceList", "getDigInputs", "getDigOutputs", "getDriverPowerStatus", "getFirmwareVer", "getHighSpeed", "getIdleCurrent", "getLowSpeed", "getMode", "getPolarity", "getPosition", "getProductId", "getRunCurrent", "getStatus", "homeMotorNeg", "homeMotorPos", "initialize", "jogConstNeg", "jogConstPos", "moveToPos", "openRef", "pause", "powerOFF", "powerON", "processEvents", "rawCmd", "setAcceleration", "setDeviceId", "setDigOutput", "setHighSpeed", "setLowSpeed", "setPolarity", "setPosition", "setRunCurrent", "setIdleCurrent", "setMode", "setTimeOuts", "stopImmediately", "stopSlowly", "storeToFlashMem", "updatePanelItems", "validateDemoPos", "validatePos", "waitUntilDone", "zeroPosition"] ("actions")
                  }
                }
              }
              event "high_speed_set": Value Change {
                w355 = T7[] [enum."setHighSpeed", enum."processEvents"] items=["------- unused -------", "about", "checkModel", "clearError", "closeRef", "demo", "getAcceleration", "getActualCurrentVal", "getDeviceId", "getDeviceList", "getDigInputs", "getDigOutputs", "getDriverPowerStatus", "getFirmwareVer", "getHighSpeed", "getIdleCurrent", "getLowSpeed", "getMode", "getPolarity", "getPosition", "getProductId", "getRunCurrent", "getStatus", "homeMotorNeg", "homeMotorPos", "initialize", "jogConstNeg", "jogConstPos", "moveToPos", "openRef", "pause", "powerOFF", "powerON", "processEvents", "rawCmd", "setAcceleration", "setDeviceId", "setDigOutput", "setHighSpeed", "setLowSpeed", "setPolarity", "setPosition", "setRunCurrent", "setIdleCurrent", "setMode", "setTimeOuts", "stopImmediately", "stopSlowly", "storeToFlashMem", "updatePanelItems", "validateDemoPos", "validatePos", "waitUntilDone", "zeroPosition"] ("actions")
                n130 = event-data() -> ()  [unwired: 1 in, 6 out]
              }
              event "low_speed_set": Value Change {
                w357 = T7[] [enum."setLowSpeed", enum."processEvents"] items=["------- unused -------", "about", "checkModel", "clearError", "closeRef", "demo", "getAcceleration", "getActualCurrentVal", "getDeviceId", "getDeviceList", "getDigInputs", "getDigOutputs", "getDriverPowerStatus", "getFirmwareVer", "getHighSpeed", "getIdleCurrent", "getLowSpeed", "getMode", "getPolarity", "getPosition", "getProductId", "getRunCurrent", "getStatus", "homeMotorNeg", "homeMotorPos", "initialize", "jogConstNeg", "jogConstPos", "moveToPos", "openRef", "pause", "powerOFF", "powerON", "processEvents", "rawCmd", "setAcceleration", "setDeviceId", "setDigOutput", "setHighSpeed", "setLowSpeed", "setPolarity", "setPosition", "setRunCurrent", "setIdleCurrent", "setMode", "setTimeOuts", "stopImmediately", "stopSlowly", "storeToFlashMem", "updatePanelItems", "validateDemoPos", "validatePos", "waitUntilDone", "zeroPosition"] ("actions")
                n131 = event-data() -> ()  [unwired: 1 in, 6 out]
              }
              event "accel_set": Value Change {
                w359 = T7[] [enum."setAcceleration", enum."processEvents"] items=["------- unused -------", "about", "checkModel", "clearError", "closeRef", "demo", "getAcceleration", "getActualCurrentVal", "getDeviceId", "getDeviceList", "getDigInputs", "getDigOutputs", "getDriverPowerStatus", "getFirmwareVer", "getHighSpeed", "getIdleCurrent", "getLowSpeed", "getMode", "getPolarity", "getPosition", "getProductId", "getRunCurrent", "getStatus", "homeMotorNeg", "homeMotorPos", "initialize", "jogConstNeg", "jogConstPos", "moveToPos", "openRef", "pause", "powerOFF", "powerON", "processEvents", "rawCmd", "setAcceleration", "setDeviceId", "setDigOutput", "setHighSpeed", "setLowSpeed", "setPolarity", "setPosition", "setRunCurrent", "setIdleCurrent", "setMode", "setTimeOuts", "stopImmediately", "stopSlowly", "storeToFlashMem", "updatePanelItems", "validateDemoPos", "validatePos", "waitUntilDone", "zeroPosition"] ("actions")
                n132 = event-data() -> ()  [unwired: 1 in, 6 out]
              }
              event "clear": Value Change {
                w361 = T7[] [enum."clearError", enum."processEvents"] items=["------- unused -------", "about", "checkModel", "clearError", "closeRef", "demo", "getAcceleration", "getActualCurrentVal", "getDeviceId", "getDeviceList", "getDigInputs", "getDigOutputs", "getDriverPowerStatus", "getFirmwareVer", "getHighSpeed", "getIdleCurrent", "getLowSpeed", "getMode", "getPolarity", "getPosition", "getProductId", "getRunCurrent", "getStatus", "homeMotorNeg", "homeMotorPos", "initialize", "jogConstNeg", "jogConstPos", "moveToPos", "openRef", "pause", "powerOFF", "powerON", "processEvents", "rawCmd", "setAcceleration", "setDeviceId", "setDigOutput", "setHighSpeed", "setLowSpeed", "setPolarity", "setPosition", "setRunCurrent", "setIdleCurrent", "setMode", "setTimeOuts", "stopImmediately", "stopSlowly", "storeToFlashMem", "updatePanelItems", "validateDemoPos", "validatePos", "waitUntilDone", "zeroPosition"] ("actions")
                n133 = event-data() -> ()  [unwired: 1 in, 6 out]
              }
              event "home_pos": Value Change {
                w363 = T7[] [enum."homeMotorPos", enum."processEvents"] items=["------- unused -------", "about", "checkModel", "clearError", "closeRef", "demo", "getAcceleration", "getActualCurrentVal", "getDeviceId", "getDeviceList", "getDigInputs", "getDigOutputs", "getDriverPowerStatus", "getFirmwareVer", "getHighSpeed", "getIdleCurrent", "getLowSpeed", "getMode", "getPolarity", "getPosition", "getProductId", "getRunCurrent", "getStatus", "homeMotorNeg", "homeMotorPos", "initialize", "jogConstNeg", "jogConstPos", "moveToPos", "openRef", "pause", "powerOFF", "powerON", "processEvents", "rawCmd", "setAcceleration", "setDeviceId", "setDigOutput", "setHighSpeed", "setLowSpeed", "setPolarity", "setPosition", "setRunCurrent", "setIdleCurrent", "setMode", "setTimeOuts", "stopImmediately", "stopSlowly", "storeToFlashMem", "updatePanelItems", "validateDemoPos", "validatePos", "waitUntilDone", "zeroPosition"] ("actions")
                n134 = event-data() -> ()  [unwired: 1 in, 6 out]
              }
              event "home_neg": Value Change {
                w365 = T7[] [enum."homeMotorNeg", enum."processEvents"] items=["------- unused -------", "about", "checkModel", "clearError", "closeRef", "demo", "getAcceleration", "getActualCurrentVal", "getDeviceId", "getDeviceList", "getDigInputs", "getDigOutputs", "getDriverPowerStatus", "getFirmwareVer", "getHighSpeed", "getIdleCurrent", "getLowSpeed", "getMode", "getPolarity", "getPosition", "getProductId", "getRunCurrent", "getStatus", "homeMotorNeg", "homeMotorPos", "initialize", "jogConstNeg", "jogConstPos", "moveToPos", "openRef", "pause", "powerOFF", "powerON", "processEvents", "rawCmd", "setAcceleration", "setDeviceId", "setDigOutput", "setHighSpeed", "setLowSpeed", "setPolarity", "setPosition", "setRunCurrent", "setIdleCurrent", "setMode", "setTimeOuts", "stopImmediately", "stopSlowly", "storeToFlashMem", "updatePanelItems", "validateDemoPos", "validatePos", "waitUntilDone", "zeroPosition"] ("actions")
                n135 = event-data() -> ()  [unwired: 1 in, 6 out]
              }
              event "position_val_set": Value Change {
                w367 = T7[] [enum."setPosition", enum."processEvents"] items=["------- unused -------", "about", "checkModel", "clearError", "closeRef", "demo", "getAcceleration", "getActualCurrentVal", "getDeviceId", "getDeviceList", "getDigInputs", "getDigOutputs", "getDriverPowerStatus", "getFirmwareVer", "getHighSpeed", "getIdleCurrent", "getLowSpeed", "getMode", "getPolarity", "getPosition", "getProductId", "getRunCurrent", "getStatus", "homeMotorNeg", "homeMotorPos", "initialize", "jogConstNeg", "jogConstPos", "moveToPos", "openRef", "pause", "powerOFF", "powerON", "processEvents", "rawCmd", "setAcceleration", "setDeviceId", "setDigOutput", "setHighSpeed", "setLowSpeed", "setPolarity", "setPosition", "setRunCurrent", "setIdleCurrent", "setMode", "setTimeOuts", "stopImmediately", "stopSlowly", "storeToFlashMem", "updatePanelItems", "validateDemoPos", "validatePos", "waitUntilDone", "zeroPosition"] ("actions")
                n136 = event-data() -> ()  [unwired: 1 in, 6 out]
              }
              event "demo_start": Value Change {
                n137 = event-data() -> ()  [unwired: 1 in, 6 out]
                n138 = case shown="True" "zero" {
                  tunnel: [w372 w373] -> w370
                  frame True {
                    w372 = T7[] [enum."zeroPosition", enum."demo", enum."processEvents"] items=["------- unused -------", "about", "checkModel", "clearError", "closeRef", "demo", "getAcceleration", "getActualCurrentVal", "getDeviceId", "getDeviceList", "getDigInputs", "getDigOutputs", "getDriverPowerStatus", "getFirmwareVer", "getHighSpeed", "getIdleCurrent", "getLowSpeed", "getMode", "getPolarity", "getPosition", "getProductId", "getRunCurrent", "getStatus", "homeMotorNeg", "homeMotorPos", "initialize", "jogConstNeg", "jogConstPos", "moveToPos", "openRef", "pause", "powerOFF", "powerON", "processEvents", "rawCmd", "setAcceleration", "setDeviceId", "setDigOutput", "setHighSpeed", "setLowSpeed", "setPolarity", "setPosition", "setRunCurrent", "setIdleCurrent", "setMode", "setTimeOuts", "stopImmediately", "stopSlowly", "storeToFlashMem", "updatePanelItems", "validateDemoPos", "validatePos", "waitUntilDone", "zeroPosition"] ("actions")
                  }
                  frame False {
                    w373 = T7[] [enum."demo", enum."processEvents"] items=["------- unused -------", "about", "checkModel", "clearError", "closeRef", "demo", "getAcceleration", "getActualCurrentVal", "getDeviceId", "getDeviceList", "getDigInputs", "getDigOutputs", "getDriverPowerStatus", "getFirmwareVer", "getHighSpeed", "getIdleCurrent", "getLowSpeed", "getMode", "getPolarity", "getPosition", "getProductId", "getRunCurrent", "getStatus", "homeMotorNeg", "homeMotorPos", "initialize", "jogConstNeg", "jogConstPos", "moveToPos", "openRef", "pause", "powerOFF", "powerON", "processEvents", "rawCmd", "setAcceleration", "setDeviceId", "setDigOutput", "setHighSpeed", "setLowSpeed", "setPolarity", "setPosition", "setRunCurrent", "setIdleCurrent", "setMode", "setTimeOuts", "stopImmediately", "stopSlowly", "storeToFlashMem", "updatePanelItems", "validateDemoPos", "validatePos", "waitUntilDone", "zeroPosition"] ("actions")
                  }
                }
              }
              event "move_to": Value Change {
                w374 = T7[] [enum."validatePos", enum."moveToPos", enum."processEvents"] items=["------- unused -------", "about", "checkModel", "clearError", "closeRef", "demo", "getAcceleration", "getActualCurrentVal", "getDeviceId", "getDeviceList", "getDigInputs", "getDigOutputs", "getDriverPowerStatus", "getFirmwareVer", "getHighSpeed", "getIdleCurrent", "getLowSpeed", "getMode", "getPolarity", "getPosition", "getProductId", "getRunCurrent", "getStatus", "homeMotorNeg", "homeMotorPos", "initialize", "jogConstNeg", "jogConstPos", "moveToPos", "openRef", "pause", "powerOFF", "powerON", "processEvents", "rawCmd", "setAcceleration", "setDeviceId", "setDigOutput", "setHighSpeed", "setLowSpeed", "setPolarity", "setPosition", "setRunCurrent", "setIdleCurrent", "setMode", "setTimeOuts", "stopImmediately", "stopSlowly", "storeToFlashMem", "updatePanelItems", "validateDemoPos", "validatePos", "waitUntilDone", "zeroPosition"] ("actions")
                n139 = event-data() -> ()  [unwired: 1 in, 6 out]
              }
              event Menu Selection (User) {
                n140 = event-data() -> ("ItemTag"=w379:string)  [unwired: 1 in, 6 out]
                n141 = To Lower Case(string=w379) -> (all lower case string=w378:string)
                n142 = case shown="\"toggle on/off\"" w378 {
                  selector: w378 -> [_ _ _ _ _ _ _ _ _ _ _ w396]
                  tunnel: [w380 w382 w383 w384 w385 w387 w388 w389 w390 w391 w393 w399] -> w377
                  frame "about" {
                    w380 = T7[] [enum."about", enum."processEvents"] items=["------- unused -------", "about", "checkModel", "clearError", "closeRef", "demo", "getAcceleration", "getActualCurrentVal", "getDeviceId", "getDeviceList", "getDigInputs", "getDigOutputs", "getDriverPowerStatus", "getFirmwareVer", "getHighSpeed", "getIdleCurrent", "getLowSpeed", "getMode", "getPolarity", "getPosition", "getProductId", "getRunCurrent", "getStatus", "homeMotorNeg", "homeMotorPos", "initialize", "jogConstNeg", "jogConstPos", "moveToPos", "openRef", "pause", "powerOFF", "powerON", "processEvents", "rawCmd", "setAcceleration", "setDeviceId", "setDigOutput", "setHighSpeed", "setLowSpeed", "setPolarity", "setPosition", "setRunCurrent", "setIdleCurrent", "setMode", "setTimeOuts", "stopImmediately", "stopSlowly", "storeToFlashMem", "updatePanelItems", "validateDemoPos", "validatePos", "waitUntilDone", "zeroPosition"] ("actions")
                  }
                  frame "absolute" {
                    w382 = T7[] [enum."setMode", enum."processEvents"] items=["------- unused -------", "about", "checkModel", "clearError", "closeRef", "demo", "getAcceleration", "getActualCurrentVal", "getDeviceId", "getDeviceList", "getDigInputs", "getDigOutputs", "getDriverPowerStatus", "getFirmwareVer", "getHighSpeed", "getIdleCurrent", "getLowSpeed", "getMode", "getPolarity", "getPosition", "getProductId", "getRunCurrent", "getStatus", "homeMotorNeg", "homeMotorPos", "initialize", "jogConstNeg", "jogConstPos", "moveToPos", "openRef", "pause", "powerOFF", "powerON", "processEvents", "rawCmd", "setAcceleration", "setDeviceId", "setDigOutput", "setHighSpeed", "setLowSpeed", "setPolarity", "setPosition", "setRunCurrent", "setIdleCurrent", "setMode", "setTimeOuts", "stopImmediately", "stopSlowly", "storeToFlashMem", "updatePanelItems", "validateDemoPos", "validatePos", "waitUntilDone", "zeroPosition"] ("actions")
                    n143 = local write "move_mode"(enum32{"Abs:", "Inc:"}."Abs:" ("move_mode")) -> ()
                  }
                  frame "exit" {
                    w383 = T7[] [enum."powerOFF", enum."closeRef"] items=["------- unused -------", "about", "checkModel", "clearError", "closeRef", "demo", "getAcceleration", "getActualCurrentVal", "getDeviceId", "getDeviceList", "getDigInputs", "getDigOutputs", "getDriverPowerStatus", "getFirmwareVer", "getHighSpeed", "getIdleCurrent", "getLowSpeed", "getMode", "getPolarity", "getPosition", "getProductId", "getRunCurrent", "getStatus", "homeMotorNeg", "homeMotorPos", "initialize", "jogConstNeg", "jogConstPos", "moveToPos", "openRef", "pause", "powerOFF", "powerON", "processEvents", "rawCmd", "setAcceleration", "setDeviceId", "setDigOutput", "setHighSpeed", "setLowSpeed", "setPolarity", "setPosition", "setRunCurrent", "setIdleCurrent", "setMode", "setTimeOuts", "stopImmediately", "stopSlowly", "storeToFlashMem", "updatePanelItems", "validateDemoPos", "validatePos", "waitUntilDone", "zeroPosition"] ("actions")
                  }
                  frame "home (+)" {
                    w384 = T7[] [enum."homeMotorPos", enum."processEvents"] items=["------- unused -------", "about", "checkModel", "clearError", "closeRef", "demo", "getAcceleration", "getActualCurrentVal", "getDeviceId", "getDeviceList", "getDigInputs", "getDigOutputs", "getDriverPowerStatus", "getFirmwareVer", "getHighSpeed", "getIdleCurrent", "getLowSpeed", "getMode", "getPolarity", "getPosition", "getProductId", "getRunCurrent", "getStatus", "homeMotorNeg", "homeMotorPos", "initialize", "jogConstNeg", "jogConstPos", "moveToPos", "openRef", "pause", "powerOFF", "powerON", "processEvents", "rawCmd", "setAcceleration", "setDeviceId", "setDigOutput", "setHighSpeed", "setLowSpeed", "setPolarity", "setPosition", "setRunCurrent", "setIdleCurrent", "setMode", "setTimeOuts", "stopImmediately", "stopSlowly", "storeToFlashMem", "updatePanelItems", "validateDemoPos", "validatePos", "waitUntilDone", "zeroPosition"] ("actions")
                  }
                  frame "home (-)" {
                    w385 = T7[] [enum."homeMotorNeg", enum."processEvents"] items=["------- unused -------", "about", "checkModel", "clearError", "closeRef", "demo", "getAcceleration", "getActualCurrentVal", "getDeviceId", "getDeviceList", "getDigInputs", "getDigOutputs", "getDriverPowerStatus", "getFirmwareVer", "getHighSpeed", "getIdleCurrent", "getLowSpeed", "getMode", "getPolarity", "getPosition", "getProductId", "getRunCurrent", "getStatus", "homeMotorNeg", "homeMotorPos", "initialize", "jogConstNeg", "jogConstPos", "moveToPos", "openRef", "pause", "powerOFF", "powerON", "processEvents", "rawCmd", "setAcceleration", "setDeviceId", "setDigOutput", "setHighSpeed", "setLowSpeed", "setPolarity", "setPosition", "setRunCurrent", "setIdleCurrent", "setMode", "setTimeOuts", "stopImmediately", "stopSlowly", "storeToFlashMem", "updatePanelItems", "validateDemoPos", "validatePos", "waitUntilDone", "zeroPosition"] ("actions")
                  }
                  frame "incremental" {
                    w387 = T7[] [enum."setMode", enum."processEvents"] items=["------- unused -------", "about", "checkModel", "clearError", "closeRef", "demo", "getAcceleration", "getActualCurrentVal", "getDeviceId", "getDeviceList", "getDigInputs", "getDigOutputs", "getDriverPowerStatus", "getFirmwareVer", "getHighSpeed", "getIdleCurrent", "getLowSpeed", "getMode", "getPolarity", "getPosition", "getProductId", "getRunCurrent", "getStatus", "homeMotorNeg", "homeMotorPos", "initialize", "jogConstNeg", "jogConstPos", "moveToPos", "openRef", "pause", "powerOFF", "powerON", "processEvents", "rawCmd", "setAcceleration", "setDeviceId", "setDigOutput", "setHighSpeed", "setLowSpeed", "setPolarity", "setPosition", "setRunCurrent", "setIdleCurrent", "setMode", "setTimeOuts", "stopImmediately", "stopSlowly", "storeToFlashMem", "updatePanelItems", "validateDemoPos", "validatePos", "waitUntilDone", "zeroPosition"] ("actions")
                    n144 = local write "move_mode"(enum32{"Abs:", "Inc:"}."Inc:" ("move_mode")) -> ()
                  }
                  frame "jog (+)" {
                    w388 = T7[] [enum."jogConstPos", enum."processEvents"] items=["------- unused -------", "about", "checkModel", "clearError", "closeRef", "demo", "getAcceleration", "getActualCurrentVal", "getDeviceId", "getDeviceList", "getDigInputs", "getDigOutputs", "getDriverPowerStatus", "getFirmwareVer", "getHighSpeed", "getIdleCurrent", "getLowSpeed", "getMode", "getPolarity", "getPosition", "getProductId", "getRunCurrent", "getStatus", "homeMotorNeg", "homeMotorPos", "initialize", "jogConstNeg", "jogConstPos", "moveToPos", "openRef", "pause", "powerOFF", "powerON", "processEvents", "rawCmd", "setAcceleration", "setDeviceId", "setDigOutput", "setHighSpeed", "setLowSpeed", "setPolarity", "setPosition", "setRunCurrent", "setIdleCurrent", "setMode", "setTimeOuts", "stopImmediately", "stopSlowly", "storeToFlashMem", "updatePanelItems", "validateDemoPos", "validatePos", "waitUntilDone", "zeroPosition"] ("actions")
                  }
                  frame "jog (-)" {
                    w389 = T7[] [enum."jogConstNeg", enum."processEvents"] items=["------- unused -------", "about", "checkModel", "clearError", "closeRef", "demo", "getAcceleration", "getActualCurrentVal", "getDeviceId", "getDeviceList", "getDigInputs", "getDigOutputs", "getDriverPowerStatus", "getFirmwareVer", "getHighSpeed", "getIdleCurrent", "getLowSpeed", "getMode", "getPolarity", "getPosition", "getProductId", "getRunCurrent", "getStatus", "homeMotorNeg", "homeMotorPos", "initialize", "jogConstNeg", "jogConstPos", "moveToPos", "openRef", "pause", "powerOFF", "powerON", "processEvents", "rawCmd", "setAcceleration", "setDeviceId", "setDigOutput", "setHighSpeed", "setLowSpeed", "setPolarity", "setPosition", "setRunCurrent", "setIdleCurrent", "setMode", "setTimeOuts", "stopImmediately", "stopSlowly", "storeToFlashMem", "updatePanelItems", "validateDemoPos", "validatePos", "waitUntilDone", "zeroPosition"] ("actions")
                  }
                  frame "stop quick" {
                    w390 = T7[] [enum."stopImmediately", enum."processEvents"] items=["------- unused -------", "about", "checkModel", "clearError", "closeRef", "demo", "getAcceleration", "getActualCurrentVal", "getDeviceId", "getDeviceList", "getDigInputs", "getDigOutputs", "getDriverPowerStatus", "getFirmwareVer", "getHighSpeed", "getIdleCurrent", "getLowSpeed", "getMode", "getPolarity", "getPosition", "getProductId", "getRunCurrent", "getStatus", "homeMotorNeg", "homeMotorPos", "initialize", "jogConstNeg", "jogConstPos", "moveToPos", "openRef", "pause", "powerOFF", "powerON", "processEvents", "rawCmd", "setAcceleration", "setDeviceId", "setDigOutput", "setHighSpeed", "setLowSpeed", "setPolarity", "setPosition", "setRunCurrent", "setIdleCurrent", "setMode", "setTimeOuts", "stopImmediately", "stopSlowly", "storeToFlashMem", "updatePanelItems", "validateDemoPos", "validatePos", "waitUntilDone", "zeroPosition"] ("actions")
                  }
                  frame "stop slow" {
                    w391 = T7[] [enum."stopSlowly", enum."processEvents"] items=["------- unused -------", "about", "checkModel", "clearError", "closeRef", "demo", "getAcceleration", "getActualCurrentVal", "getDeviceId", "getDeviceList", "getDigInputs", "getDigOutputs", "getDriverPowerStatus", "getFirmwareVer", "getHighSpeed", "getIdleCurrent", "getLowSpeed", "getMode", "getPolarity", "getPosition", "getProductId", "getRunCurrent", "getStatus", "homeMotorNeg", "homeMotorPos", "initialize", "jogConstNeg", "jogConstPos", "moveToPos", "openRef", "pause", "powerOFF", "powerON", "processEvents", "rawCmd", "setAcceleration", "setDeviceId", "setDigOutput", "setHighSpeed", "setLowSpeed", "setPolarity", "setPosition", "setRunCurrent", "setIdleCurrent", "setMode", "setTimeOuts", "stopImmediately", "stopSlowly", "storeToFlashMem", "updatePanelItems", "validateDemoPos", "validatePos", "waitUntilDone", "zeroPosition"] ("actions")
                  }
                  frame "toggle on/off" {
                    n145 = local read "on/off"() -> (w392:bool)
                    n146 = case shown="False" w392 {
                      tunnel: [w394 w395] -> w393
                      frame True {
                        w394 = T7[] [enum."powerOFF", enum."processEvents"] items=["------- unused -------", "about", "checkModel", "clearError", "closeRef", "demo", "getAcceleration", "getActualCurrentVal", "getDeviceId", "getDeviceList", "getDigInputs", "getDigOutputs", "getDriverPowerStatus", "getFirmwareVer", "getHighSpeed", "getIdleCurrent", "getLowSpeed", "getMode", "getPolarity", "getPosition", "getProductId", "getRunCurrent", "getStatus", "homeMotorNeg", "homeMotorPos", "initialize", "jogConstNeg", "jogConstPos", "moveToPos", "openRef", "pause", "powerOFF", "powerON", "processEvents", "rawCmd", "setAcceleration", "setDeviceId", "setDigOutput", "setHighSpeed", "setLowSpeed", "setPolarity", "setPosition", "setRunCurrent", "setIdleCurrent", "setMode", "setTimeOuts", "stopImmediately", "stopSlowly", "storeToFlashMem", "updatePanelItems", "validateDemoPos", "validatePos", "waitUntilDone", "zeroPosition"] ("actions")
                      }
                      frame False {
                        w395 = T7[] [enum."powerON", enum."processEvents"] items=["------- unused -------", "about", "checkModel", "clearError", "closeRef", "demo", "getAcceleration", "getActualCurrentVal", "getDeviceId", "getDeviceList", "getDigInputs", "getDigOutputs", "getDriverPowerStatus", "getFirmwareVer", "getHighSpeed", "getIdleCurrent", "getLowSpeed", "getMode", "getPolarity", "getPosition", "getProductId", "getRunCurrent", "getStatus", "homeMotorNeg", "homeMotorPos", "initialize", "jogConstNeg", "jogConstPos", "moveToPos", "openRef", "pause", "powerOFF", "powerON", "processEvents", "rawCmd", "setAcceleration", "setDeviceId", "setDigOutput", "setHighSpeed", "setLowSpeed", "setPolarity", "setPosition", "setRunCurrent", "setIdleCurrent", "setMode", "setTimeOuts", "stopImmediately", "stopSlowly", "storeToFlashMem", "updatePanelItems", "validateDemoPos", "validatePos", "waitUntilDone", "zeroPosition"] ("actions")
                      }
                    }
                  }
                  frame Default {
                    w399 = T7[] [enum."processEvents"] items=["------- unused -------", "about", "checkModel", "clearError", "closeRef", "demo", "getAcceleration", "getActualCurrentVal", "getDeviceId", "getDeviceList", "getDigInputs", "getDigOutputs", "getDriverPowerStatus", "getFirmwareVer", "getHighSpeed", "getIdleCurrent", "getLowSpeed", "getMode", "getPolarity", "getPosition", "getProductId", "getRunCurrent", "getStatus", "homeMotorNeg", "homeMotorPos", "initialize", "jogConstNeg", "jogConstPos", "moveToPos", "openRef", "pause", "powerOFF", "powerON", "processEvents", "rawCmd", "setAcceleration", "setDeviceId", "setDigOutput", "setHighSpeed", "setLowSpeed", "setPolarity", "setPosition", "setRunCurrent", "setIdleCurrent", "setMode", "setTimeOuts", "stopImmediately", "stopSlowly", "storeToFlashMem", "updatePanelItems", "validateDemoPos", "validatePos", "waitUntilDone", "zeroPosition"] ("actions")
                    n147 = Format Into String(format string="Unknown Menu Item '%s'" ("message"), w396) -> (resulting string=w397:string)  [unwired: 2 in, 1 out]
                    n148 = One Button Dialog(message=w397) -> ()  [unwired: 1 in, 1 out]
                  }
                }
              }
              event "polarities": Value Change {
                w400 = T7[] [enum."setPolarity", enum."processEvents"] items=["------- unused -------", "about", "checkModel", "clearError", "closeRef", "demo", "getAcceleration", "getActualCurrentVal", "getDeviceId", "getDeviceList", "getDigInputs", "getDigOutputs", "getDriverPowerStatus", "getFirmwareVer", "getHighSpeed", "getIdleCurrent", "getLowSpeed", "getMode", "getPolarity", "getPosition", "getProductId", "getRunCurrent", "getStatus", "homeMotorNeg", "homeMotorPos", "initialize", "jogConstNeg", "jogConstPos", "moveToPos", "openRef", "pause", "powerOFF", "powerON", "processEvents", "rawCmd", "setAcceleration", "setDeviceId", "setDigOutput", "setHighSpeed", "setLowSpeed", "setPolarity", "setPosition", "setRunCurrent", "setIdleCurrent", "setMode", "setTimeOuts", "stopImmediately", "stopSlowly", "storeToFlashMem", "updatePanelItems", "validateDemoPos", "validatePos", "waitUntilDone", "zeroPosition"] ("actions")
                n149 = event-data() -> ()  [unwired: 1 in, 6 out]
              }
              event "help": Value Change {
                w404 = T7[] [enum."processEvents"] items=["------- unused -------", "about", "checkModel", "clearError", "closeRef", "demo", "getAcceleration", "getActualCurrentVal", "getDeviceId", "getDeviceList", "getDigInputs", "getDigOutputs", "getDriverPowerStatus", "getFirmwareVer", "getHighSpeed", "getIdleCurrent", "getLowSpeed", "getMode", "getPolarity", "getPosition", "getProductId", "getRunCurrent", "getStatus", "homeMotorNeg", "homeMotorPos", "initialize", "jogConstNeg", "jogConstPos", "moveToPos", "openRef", "pause", "powerOFF", "powerON", "processEvents", "rawCmd", "setAcceleration", "setDeviceId", "setDigOutput", "setHighSpeed", "setLowSpeed", "setPolarity", "setPosition", "setRunCurrent", "setIdleCurrent", "setMode", "setTimeOuts", "stopImmediately", "stopSlowly", "storeToFlashMem", "updatePanelItems", "validateDemoPos", "validatePos", "waitUntilDone", "zeroPosition"] ("actions")
                n150 = event-data() -> ()  [unwired: 1 in, 6 out]
                n151 = fn#1354() -> (1:w403:bool)  [unwired: 1 out]
                n152 = Not(x=w403) -> (.not. x?=w402:bool)
                n153 = Control Help Window(1:w402) -> ()  [unwired: 1 in]
              }
              event "dig_outs", "polarities.Digital Output": Value Change {
                w406 = T7[] [enum."setDigOutput", enum."processEvents"] items=["------- unused -------", "about", "checkModel", "clearError", "closeRef", "demo", "getAcceleration", "getActualCurrentVal", "getDeviceId", "getDeviceList", "getDigInputs", "getDigOutputs", "getDriverPowerStatus", "getFirmwareVer", "getHighSpeed", "getIdleCurrent", "getLowSpeed", "getMode", "getPolarity", "getPosition", "getProductId", "getRunCurrent", "getStatus", "homeMotorNeg", "homeMotorPos", "initialize", "jogConstNeg", "jogConstPos", "moveToPos", "openRef", "pause", "powerOFF", "powerON", "processEvents", "rawCmd", "setAcceleration", "setDeviceId", "setDigOutput", "setHighSpeed", "setLowSpeed", "setPolarity", "setPosition", "setRunCurrent", "setIdleCurrent", "setMode", "setTimeOuts", "stopImmediately", "stopSlowly", "storeToFlashMem", "updatePanelItems", "validateDemoPos", "validatePos", "waitUntilDone", "zeroPosition"] ("actions")
                n154 = event-data() -> ()  [unwired: 1 in, 6 out]
              }
              event "move_mode": Value Change {
                w408 = T7[] [enum."setMode", enum."processEvents"] items=["------- unused -------", "about", "checkModel", "clearError", "closeRef", "demo", "getAcceleration", "getActualCurrentVal", "getDeviceId", "getDeviceList", "getDigInputs", "getDigOutputs", "getDriverPowerStatus", "getFirmwareVer", "getHighSpeed", "getIdleCurrent", "getLowSpeed", "getMode", "getPolarity", "getPosition", "getProductId", "getRunCurrent", "getStatus", "homeMotorNeg", "homeMotorPos", "initialize", "jogConstNeg", "jogConstPos", "moveToPos", "openRef", "pause", "powerOFF", "powerON", "processEvents", "rawCmd", "setAcceleration", "setDeviceId", "setDigOutput", "setHighSpeed", "setLowSpeed", "setPolarity", "setPosition", "setRunCurrent", "setIdleCurrent", "setMode", "setTimeOuts", "stopImmediately", "stopSlowly", "storeToFlashMem", "updatePanelItems", "validateDemoPos", "validatePos", "waitUntilDone", "zeroPosition"] ("actions")
                n155 = event-data() -> ()  [unwired: 1 in, 6 out]
              }
            }
          }
          frame "rawCmd" {
            # "avoid shutting\ndown the app\nin the event\nincorrectly \nformatted commands\nare entered."
            n156 = call "send_receive_command.vi"("reference (in)"=w412, "ASCII Command (in)"="raw_cmd", "error in (no error)"=w417) -> ("reference (out)"=w411:refnum<class "_Controller.lvclass">, "response (out)"=→"response":string)  [unwired: 12 in, 3 out]
          }
          frame "setAcceleration" {
            n157 = Format Into String(format string="ACC=%d", "accel") -> (resulting string=w418:string)  [unwired: 2 in, 1 out]
            n158 = call "send_receive_command.vi"("reference (in)"=w423, "ASCII Command (in)"=w418, "error in (no error)"=w425) -> ("reference (out)"=w422:refnum<class "_Controller.lvclass">, "error out"=w424:errorcluster)  [unwired: 12 in, 3 out]
            n159 = Build Array (concatenate)(utility_actions."getAcceleration" ("Enum"), w427) -> (w426:T7[])
          }
          frame "setDeviceId" {
            n160 = Format Into String(format string="DN=%s", "new_id") -> (resulting string=w429:string)  [unwired: 2 in, 1 out]
            n161 = call "send_receive_command.vi"("reference (in)"=w436, "ASCII Command (in)"=w429, "error in (no error)"=w437) -> ("reference (out)"=w435:refnum<class "_Controller.lvclass">, "error out"=w434:errorcluster)  [unwired: 12 in, 3 out]
            n162 = case shown="Error" w434 {
              selector: w434 -> [w442 _]
              tunnel: [w442 errorcluster {"status"=FALSE, "code"=0, "source"=""} ("error out")] -> w433
              tunnel: [w441 w443] -> w432
              frame No Error {
                w441 = T7[] [enum."getDeviceId", enum."storeToFlashMem"] items=["------- unused -------", "about", "checkModel", "clearError", "closeRef", "demo", "getAcceleration", "getActualCurrentVal", "getDeviceId", "getDeviceList", "getDigInputs", "getDigOutputs", "getDriverPowerStatus", "getFirmwareVer", "getHighSpeed", "getIdleCurrent", "getLowSpeed", "getMode", "getPolarity", "getPosition", "getProductId", "getRunCurrent", "getStatus", "homeMotorNeg", "homeMotorPos", "initialize", "jogConstNeg", "jogConstPos", "moveToPos", "openRef", "pause", "powerOFF", "powerON", "processEvents", "rawCmd", "setAcceleration", "setDeviceId", "setDigOutput", "setHighSpeed", "setLowSpeed", "setPolarity", "setPosition", "setRunCurrent", "setIdleCurrent", "setMode", "setTimeOuts", "stopImmediately", "stopSlowly", "storeToFlashMem", "updatePanelItems", "validateDemoPos", "validatePos", "waitUntilDone", "zeroPosition"]
              }
              frame Error {
                w443 = T7[] [] items=["------- unused -------", "about", "checkModel", "clearError", "closeRef", "demo", "getAcceleration", "getActualCurrentVal", "getDeviceId", "getDeviceList", "getDigInputs", "getDigOutputs", "getDriverPowerStatus", "getFirmwareVer", "getHighSpeed", "getIdleCurrent", "getLowSpeed", "getMode", "getPolarity", "getPosition", "getProductId", "getRunCurrent", "getStatus", "homeMotorNeg", "homeMotorPos", "initialize", "jogConstNeg", "jogConstPos", "moveToPos", "openRef", "pause", "powerOFF", "powerON", "processEvents", "rawCmd", "setAcceleration", "setDeviceId", "setDigOutput", "setHighSpeed", "setLowSpeed", "setPolarity", "setPosition", "setRunCurrent", "setIdleCurrent", "setMode", "setTimeOuts", "stopImmediately", "stopSlowly", "storeToFlashMem", "updatePanelItems", "validateDemoPos", "validatePos", "waitUntilDone", "zeroPosition"]
                n163 = One Button Dialog(message="An error was detected while\nattempting to change the \nDevice ID.  Please check the\nformatting of the ID and \ntry again.") -> ()  [unwired: 1 in, 1 out]
              }
            }
            n164 = Build Array (concatenate)(w432, w439) -> (w438:T7[])
          }
          frame "setDigOutput" {
            n165 = Unbundle By Name("dig_outs") -> ("Digital Output 2"=w447:bool, "Digital Output 1"=w452:bool)
            n166 = call "setDigitalOutput.vi"("Controller in"=w454, "digital_output_ch"=digital_output."DIG_OUT_1", "dig_out_value"=w452, "error in (no error)"=w455) -> ("Controller out"=w450:refnum<class "_Controller.lvclass">, "error out"=w448:errorcluster)  [unwired: 12 in, 2 out]
            n167 = call "setDigitalOutput.vi"("Controller in"=w450, "digital_output_ch"=digital_output."DIG_OUT_2", "dig_out_value"=w447, "error in (no error)"=w448) -> ("Controller out"=w449:refnum<class "_Controller.lvclass">, "error out"=w446:errorcluster)  [unwired: 12 in, 2 out]
            n168 = Build Array (concatenate)(utility_actions."getDigOutputs" ("Enum"), w459) -> (w458:T7[])
          }
          frame "setHighSpeed" {
            n169 = Format Into String(format string="HSPD=%d", "high_speed") -> (resulting string=w463:string)  [unwired: 2 in, 1 out]
            n170 = call "send_receive_command.vi"("reference (in)"=w466, "ASCII Command (in)"=w463, "error in (no error)"=w468) -> ("reference (out)"=w465:refnum<class "_Controller.lvclass">, "error out"=w467:errorcluster)  [unwired: 12 in, 3 out]
            n171 = Build Array (concatenate)(utility_actions."getHighSpeed" ("Enum"), w470) -> (w469:T7[])
          }
          frame "setLowSpeed" {
            n172 = Format Into String(format string="LSPD=%d", "low_speed") -> (resulting string=w474:string)  [unwired: 2 in, 1 out]
            n173 = call "send_receive_command.vi"("reference (in)"=w477, "ASCII Command (in)"=w474, "error in (no error)"=w479) -> ("reference (out)"=w476:refnum<class "_Controller.lvclass">, "error out"=w478:errorcluster)  [unwired: 12 in, 3 out]
            n174 = Build Array (concatenate)(utility_actions."getLowSpeed" ("Enum"), w481) -> (w480:T7[])
          }
          frame "setPolarity" {
            n175 = Cluster To Array(cluster="polarities") -> (array=w489:bool[])
            n176 = for {
              tunnel: w489 -> [w494] mode=indexing
              tunnel: T13[] [{"item"=enum."DIRECTION", "status"=FALSE}, {"item"=enum."LIMIT", "status"=FALSE}, {"item"=enum."HOME", "status"=FALSE}, {"item"=enum."DIG_OUT", "status"=FALSE}, {"item"=enum."DIG_IN", "status"=FALSE}, {"item"=enum."ENABLE_OUT", "status"=FALSE}, {"item"=enum."JUMP_ERR", "status"=FALSE}] ("polarity_items") -> [w495] mode=indexing
              tunnel: [w493] -> w483 mode=indexing
              n177 = Bundle By Name(cluster=w495, "status"=w494) -> (w493:T13)
            }
            n178 = call-dynamic "setPolarity.vi"("Controller in"=w485, "polarity_items (in)"=w483, "error in (no error)"=w487) -> ("Controller out"=w484:refnum<class "_Controller.lvclass">, "error out"=w486:errorcluster)  [unwired: 13 in, 2 out]
          }
          frame "setPosition" {
            n179 = Format Into String(format string="PX=%d", "position_val_desired") -> (resulting string=w498:string)  [unwired: 2 in, 1 out]
            n180 = call "send_receive_command.vi"("reference (in)"=w501, "ASCII Command (in)"=w498, "error in (no error)"=w503) -> ("reference (out)"=w500:refnum<class "_Controller.lvclass">, "error out"=w502:errorcluster)  [unwired: 12 in, 3 out]
            n181 = Build Array (concatenate)(utility_actions."getPosition" ("Enum"), w505) -> (w504:T7[])
          }
          frame "setRunCurrent" {
            n182 = Format Into String(format string="CUR=%d", "running_amp") -> (resulting string=w509:string)  [unwired: 2 in, 1 out]
            n183 = call "send_receive_command.vi"("reference (in)"=w512, "ASCII Command (in)"=w509, "error in (no error)"=w514) -> ("reference (out)"=w511:refnum<class "_Controller.lvclass">, "error out"=w513:errorcluster)  [unwired: 12 in, 3 out]
            n184 = Build Array (concatenate)(utility_actions."getRunCurrent" ("Enum"), w516) -> (w515:T7[])
          }
          frame "setIdleCurrent" {
            n185 = Format Into String(format string="ACR=%d", "idle_amp") -> (resulting string=w520:string)  [unwired: 2 in, 1 out]
            n186 = call "send_receive_command.vi"("reference (in)"=w523, "ASCII Command (in)"=w520, "error in (no error)"=w525) -> ("reference (out)"=w522:refnum<class "_Controller.lvclass">, "error out"=w524:errorcluster)  [unwired: 12 in, 3 out]
            n187 = Build Array (concatenate)(utility_actions."getIdleCurrent" ("Enum"), w527) -> (w526:T7[])
          }
          frame "setMode" {
            n188 = case shown="\"Abs:\"" "move_mode" {
              tunnel: [move_mode."INCREMENTAL" ("mode") move_mode."ABSOLUTE" ("mode")] -> w529
              frame "Inc:" {
              }
              frame "Abs:" {
              }
            }
            n189 = call "setMoveMode.vi"("Controller in"=w531, "mode"=w529, "error in (no error)"=w532) -> ("Controller out"=w530:refnum<class "_Controller.lvclass">, "error out"=w533:errorcluster)  [unwired: 13 in, 2 out]
            n190 = Build Array (concatenate)(utility_actions."getMode" ("Enum"), w537) -> (w536:T7[])
          }
          frame "stopImmediately" {
            w542 = u8 0 ("Disabled")
            n191 = call "send_receive_command.vi"("reference (in)"=w544, "ASCII Command (in)"="ABORT", "error in (no error)"=w546) -> ("reference (out)"=w543:refnum<class "_Controller.lvclass">, "error out"=w545:errorcluster)  [unwired: 12 in, 3 out]
            n192 = property on="home_neg" class="Bool"("Disabled"=w542) -> ()  [unwired: 2 in, 2 out]
            n193 = property on="home_pos" class="Bool"("Disabled"=w542) -> ()  [unwired: 2 in, 2 out]
            n194 = property on="move_to" class="Bool"("Disabled"=w542) -> ()  [unwired: 2 in, 2 out]
            n195 = property on="jog_pos" class="Bool"("Disabled"=w542) -> ()  [unwired: 2 in, 2 out]
            n196 = property on="jog_neg" class="Bool"("Disabled"=w542) -> ()  [unwired: 2 in, 2 out]
          }
          frame "stopSlowly" {
            w550 = u8 0 ("Disabled")
            n197 = call "send_receive_command.vi"("reference (in)"=w552, "ASCII Command (in)"="STOP", "error in (no error)"=w554) -> ("reference (out)"=w551:refnum<class "_Controller.lvclass">, "error out"=w553:errorcluster)  [unwired: 12 in, 3 out]
            n198 = property on="home_neg" class="Bool"("Disabled"=w550) -> ()  [unwired: 2 in, 2 out]
            n199 = property on="home_pos" class="Bool"("Disabled"=w550) -> ()  [unwired: 2 in, 2 out]
            n200 = property on="move_to" class="Bool"("Disabled"=w550) -> ()  [unwired: 2 in, 2 out]
            n201 = property on="jog_pos" class="Bool"("Disabled"=w550) -> ()  [unwired: 2 in, 2 out]
            n202 = property on="jog_neg" class="Bool"("Disabled"=w550) -> ()  [unwired: 2 in, 2 out]
          }
          frame "storeToFlashMem" {
            n203 = call "send_receive_command.vi"("reference (in)"=w559, "ASCII Command (in)"="STORE", "error in (no error)"=w561) -> ("reference (out)"=w558:refnum<class "_Controller.lvclass">, "error out"=w560:errorcluster)  [unwired: 12 in, 3 out]
          }
          frame "updatePanelItems" {
            w566 = T7[] [] items=["------- unused -------", "about", "checkModel", "clearError", "closeRef", "demo", "getAcceleration", "getActualCurrentVal", "getDeviceId", "getDeviceList", "getDigInputs", "getDigOutputs", "getDriverPowerStatus", "getFirmwareVer", "getHighSpeed", "getIdleCurrent", "getLowSpeed", "getMode", "getPolarity", "getPosition", "getProductId", "getRunCurrent", "getStatus", "homeMotorNeg", "homeMotorPos", "initialize", "jogConstNeg", "jogConstPos", "moveToPos", "openRef", "pause", "powerOFF", "powerON", "processEvents", "rawCmd", "setAcceleration", "setDeviceId", "setDigOutput", "setHighSpeed", "setLowSpeed", "setPolarity", "setPosition", "setRunCurrent", "setIdleCurrent", "setMode", "setTimeOuts", "stopImmediately", "stopSlowly", "storeToFlashMem", "updatePanelItems", "validateDemoPos", "validatePos", "waitUntilDone", "zeroPosition"] ("actions")
            n204 = Build Array (concatenate)(w566, w567) -> (w565:T7[])
          }
          frame "validateDemoPos" {
            w580 = 262143
            n205 = local read "position_val_actual"() -> (w588:i32)
            n206 = Add(x=w588, y=w580) -> (x+y=w587:i32)
            n207 = Subtract(x=w588, y=w580) -> (x-y=w586:i32)
            n208 = Add(x="pos_1", y=w580) -> (x+y=w584:i32)
            n209 = Subtract(x="pos_1", y=w580) -> (x-y=w585:i32)
            n210 = Add(x="pos_2", y=w580) -> (x+y=w583:i32)
            n211 = Subtract(x="pos_2", y=w580) -> (x-y=w582:i32)
            n212 = In Range and Coerce(upper limit=w587, x="pos_1", lower limit=w586) -> (In Range?=w577:bool)  [unwired: 1 out]
            n213 = In Range and Coerce(upper limit=w584, x="pos_2", lower limit=w585) -> (In Range?=w578:bool)  [unwired: 1 out]
            n214 = In Range and Coerce(upper limit=w583, x="pos_3", lower limit=w582) -> (In Range?=w576:bool)  [unwired: 1 out]
            n215 = Compound Arithmetic op=AND(w577, w578, w576) -> (w574:bool)
            n216 = case shown="False" w574 {
              tunnel: w575 -> [_ w594]
              tunnel: w572 -> [w593 w595]
              tunnel: [w593 w595] -> w573
              tunnel: [w592 w594] -> w571
              frame False {
                w592 = T7[] [enum."processEvents"] items=["------- unused -------", "about", "checkModel", "clearError", "closeRef", "demo", "getAcceleration", "getActualCurrentVal", "getDeviceId", "getDeviceList", "getDigInputs", "getDigOutputs", "getDriverPowerStatus", "getFirmwareVer", "getHighSpeed", "getIdleCurrent", "getLowSpeed", "getMode", "getPolarity", "getPosition", "getProductId", "getRunCurrent", "getStatus", "homeMotorNeg", "homeMotorPos", "initialize", "jogConstNeg", "jogConstPos", "moveToPos", "openRef", "pause", "powerOFF", "powerON", "processEvents", "rawCmd", "setAcceleration", "setDeviceId", "setDigOutput", "setHighSpeed", "setLowSpeed", "setPolarity", "setPosition", "setRunCurrent", "setIdleCurrent", "setMode", "setTimeOuts", "stopImmediately", "stopSlowly", "storeToFlashMem", "updatePanelItems", "validateDemoPos", "validatePos", "waitUntilDone", "zeroPosition"] ("actions")
                n217 = One Button Dialog(message="all position values must \nfall within +/- 262143\nticks of the previous \nposition.  Please make \nthe necessary corrections\nand try again.") -> ()  [unwired: 1 in, 1 out]
              }
              frame True {
              }
            }
          }
          frame "validatePos" {
            w602 = 262143
            n218 = local read "position_val_actual"() -> (w605:i32)
            n219 = Add(x=w605, y=w602) -> (x+y=w604:i32)
            n220 = Subtract(x=w605, y=w602) -> (x-y=w603:i32)
            n221 = In Range and Coerce(upper limit=w604, x="jog_to_pos", lower limit=w603) -> (In Range?=w596:bool)  [unwired: 1 out]
            n222 = case shown="False" w596 {
              tunnel: w601 -> [_ w611]
              tunnel: w599 -> [w610 w612]
              tunnel: [w610 w612] -> w600
              tunnel: [w609 w611] -> w598
              frame False {
                w609 = T7[] [enum."processEvents"] items=["------- unused -------", "about", "checkModel", "clearError", "closeRef", "demo", "getAcceleration", "getActualCurrentVal", "getDeviceId", "getDeviceList", "getDigInputs", "getDigOutputs", "getDriverPowerStatus", "getFirmwareVer", "getHighSpeed", "getIdleCurrent", "getLowSpeed", "getMode", "getPolarity", "getPosition", "getProductId", "getRunCurrent", "getStatus", "homeMotorNeg", "homeMotorPos", "initialize", "jogConstNeg", "jogConstPos", "moveToPos", "openRef", "pause", "powerOFF", "powerON", "processEvents", "rawCmd", "setAcceleration", "setDeviceId", "setDigOutput", "setHighSpeed", "setLowSpeed", "setPolarity", "setPosition", "setRunCurrent", "setIdleCurrent", "setMode", "setTimeOuts", "stopImmediately", "stopSlowly", "storeToFlashMem", "updatePanelItems", "validateDemoPos", "validatePos", "waitUntilDone", "zeroPosition"] ("actions")
                n223 = One Button Dialog(message="all position values must \nfall within +/- 262143\nticks of the current \nposition.  Please make \nthe necessary corrections\nand try again.") -> ()  [unwired: 1 in, 1 out]
              }
              frame True {
              }
            }
          }
          frame "zeroPosition" {
            n224 = Format Into String(format string="PX=%d", 0) -> (resulting string=w613:string)  [unwired: 2 in, 1 out]
            n225 = call "send_receive_command.vi"("reference (in)"=w618, "ASCII Command (in)"=w613, "error in (no error)"=w620) -> ("reference (out)"=w617:refnum<class "_Controller.lvclass">, "error out"=w619:errorcluster)  [unwired: 12 in, 3 out]
            n226 = Build Array (concatenate)(utility_actions."getPosition" ("Enum"), w622) -> (w621:T7[])
          }
        }
        n227 = Array Size(array=w29) -> (size(s)=w28:i32)
        n228 = Unbundle By Name(w24) -> ("status"=w26:bool)
        n229 = Equal To 0?(x=w28) -> (x = 0?=w27:bool)
        n230 = Or(x=w27, y=w26) -> (x .or. y?=w25:bool)
      }
      n231 = case shown="Error" w7 {
        selector: w7 -> [w13 w14]
        tunnel: w6 -> [_ w19]
        tunnel: [w13 w18] -> w4
        frame No Error {
        }
        frame Error {
          # "In case of unexpected\nerrors, close connection"
          n232 = Unbundle By Name(w14) -> ("source"=w16:string)
          n233 = Build Array(w16) -> (w15:string[])
          n234 = call "common_errors.vi"("common_errors"=error_actions."unknown" ("errors"), "supp_text"=w15) -> ()  [unwired: 13 in, 1 out]
          n235 = call "close_connection.vi"("reference (in)"=w19, "error in (no error)"=w14) -> ("error out"=w18:errorcluster)  [unwired: 16 in, 1 out]
        }
      }
      n236 = flat-sequence {
        tunnel: w4 -> [w10]
        tunnel: [w10] -> w3
        frame #0 {
          n237 = Current VI's Path() -> (path=w12:path)
          n238 = call "get_exe_home_path.vi"("home_path"=w12) -> ("running in an executable?"=w11:bool)  [unwired: 6 in, 1 out]
          n239 = Quit LabVIEW(quit? (T)=w11) -> ()
        }
      }
    }
    frame Error {
    }
  }
  "error out" <- w1
